vi "Oscilloscope.vi"() -> ()   [LabVIEW 2018]
uses:
  NetworkStream/NetworkStreamReceiverState.ctl
  Read and Save Files/VIstatus.ctl
  NetworkStream/NetworkStreamStateMachineVariable.ctl
  NetworkStream/NetworkStreamData.ctl
  Shared program Control/MasterStatus.ctl
  <vilib>/dex/Stream Element Allocation Mode.ctl
  Read and Save Files/RW_Protocols.lvlib
  NetworkStream/NetworkStream.lvlib
  Shared program Control/MySharedVariables.lvlib
  Tektronik3102/GageNetwork.lvlib
panel:
  out "size(s)":i32[](array[numeric])
  out "loop status":T1
  out "Sequence Number":i64
  out "sequence number":u64
  out "Session Hash":u64
  out "Network Stream State Indicator":T2
  in  "Save Loop acquire":bool
  out "error out 2":errorcluster
  in  "loop acquire":bool
  in  "Tab Control 2":enum32{"single acquire", "sequence acquire"}(tab)
  out "Waveform Graph":dbl[][](graph)
  out "Intensity Chart":dbl[][](graph)
  out "aquire time (ms)":u32
  out "current aquisition":T3
  in  "abort aquisition":bool
  out "Handle Cluster":T4
  out "Gage progess":string
  in  "aquire":bool
  in  "Stop Button":bool
  out "error out":errorcluster
  in  "Tab Control":T5(tab)
  in  "channels \nconfiguration":T6(array[cluster])=[{"Coupling"=0, "Differential Input"=FALSE, "Direct-to-ADC"=FALSE, "Range"=2000, "Impedance"=50, "DC Offset"=0}, {"Coupling"=0, "Differential Input"=FALSE, "Direct-to-ADC"=FALSE, "Range"=2000, "Impedance"=50, "DC Offset"=0}, {"Coupling"=0, "Differential Input"=FALSE, "Direct-to-ADC"=FALSE, "Range"=2000, "Impedance"=50, "DC Offset"=0}, {"Coupling"=0, "Differential Input"=FALSE, "Direct-to-ADC"=FALSE, "Range"=2000, "Impedance"=50, "DC Offset"=0}] {"Impedance" min=50 max=1000000 step=999950; "Coupling" items=["DC", "AC"]}
  in  "Continuous":bool
  in  "Trigger":T7={"Slope"=0, "Level"=0, "Source"=0, "External Range"=2000, "External Coupling"=0, "External"=FALSE, "Disable"=FALSE, "External Impedance"=1} {"External Impedance" items=["50 Ohm", "HiZ"]; "External Coupling" items=["DC", "AC"]; "External Range" min=2000 max=10000 step=8000; "Slope" items=["Rising", "Falling"]; "Level" min=-100 max=100; "Source" min=0 max=64 step=1}
  in  "Acquisition":T8={"Sample Rate"=1000000.0, "Clock mode"=enum."Internal", "Mode"=0, "post trigger"=8192.0, "Segment Size"=8192.0, "Trigger Timeout"=100000.0, "Trigger Holdoff"=0.0, "Trigger Delay"=0.0, "averaging "=1} {"Segment Size" min=256.0 step=128.0; "Trigger Holdoff" min=0.0 step=128.0; "Trigger Delay" min=0.0 step=128.0; "post trigger" min=256.0 step=128.0; "Mode" items=["Single", "Dual", "Quad", "Octal"]}
  in  "configure":bool
  in  "saving folder":path=path "D:/Data/Mai/test target/logfile"
  in  "file name":string
  out "System:":string
  out "system information":T9
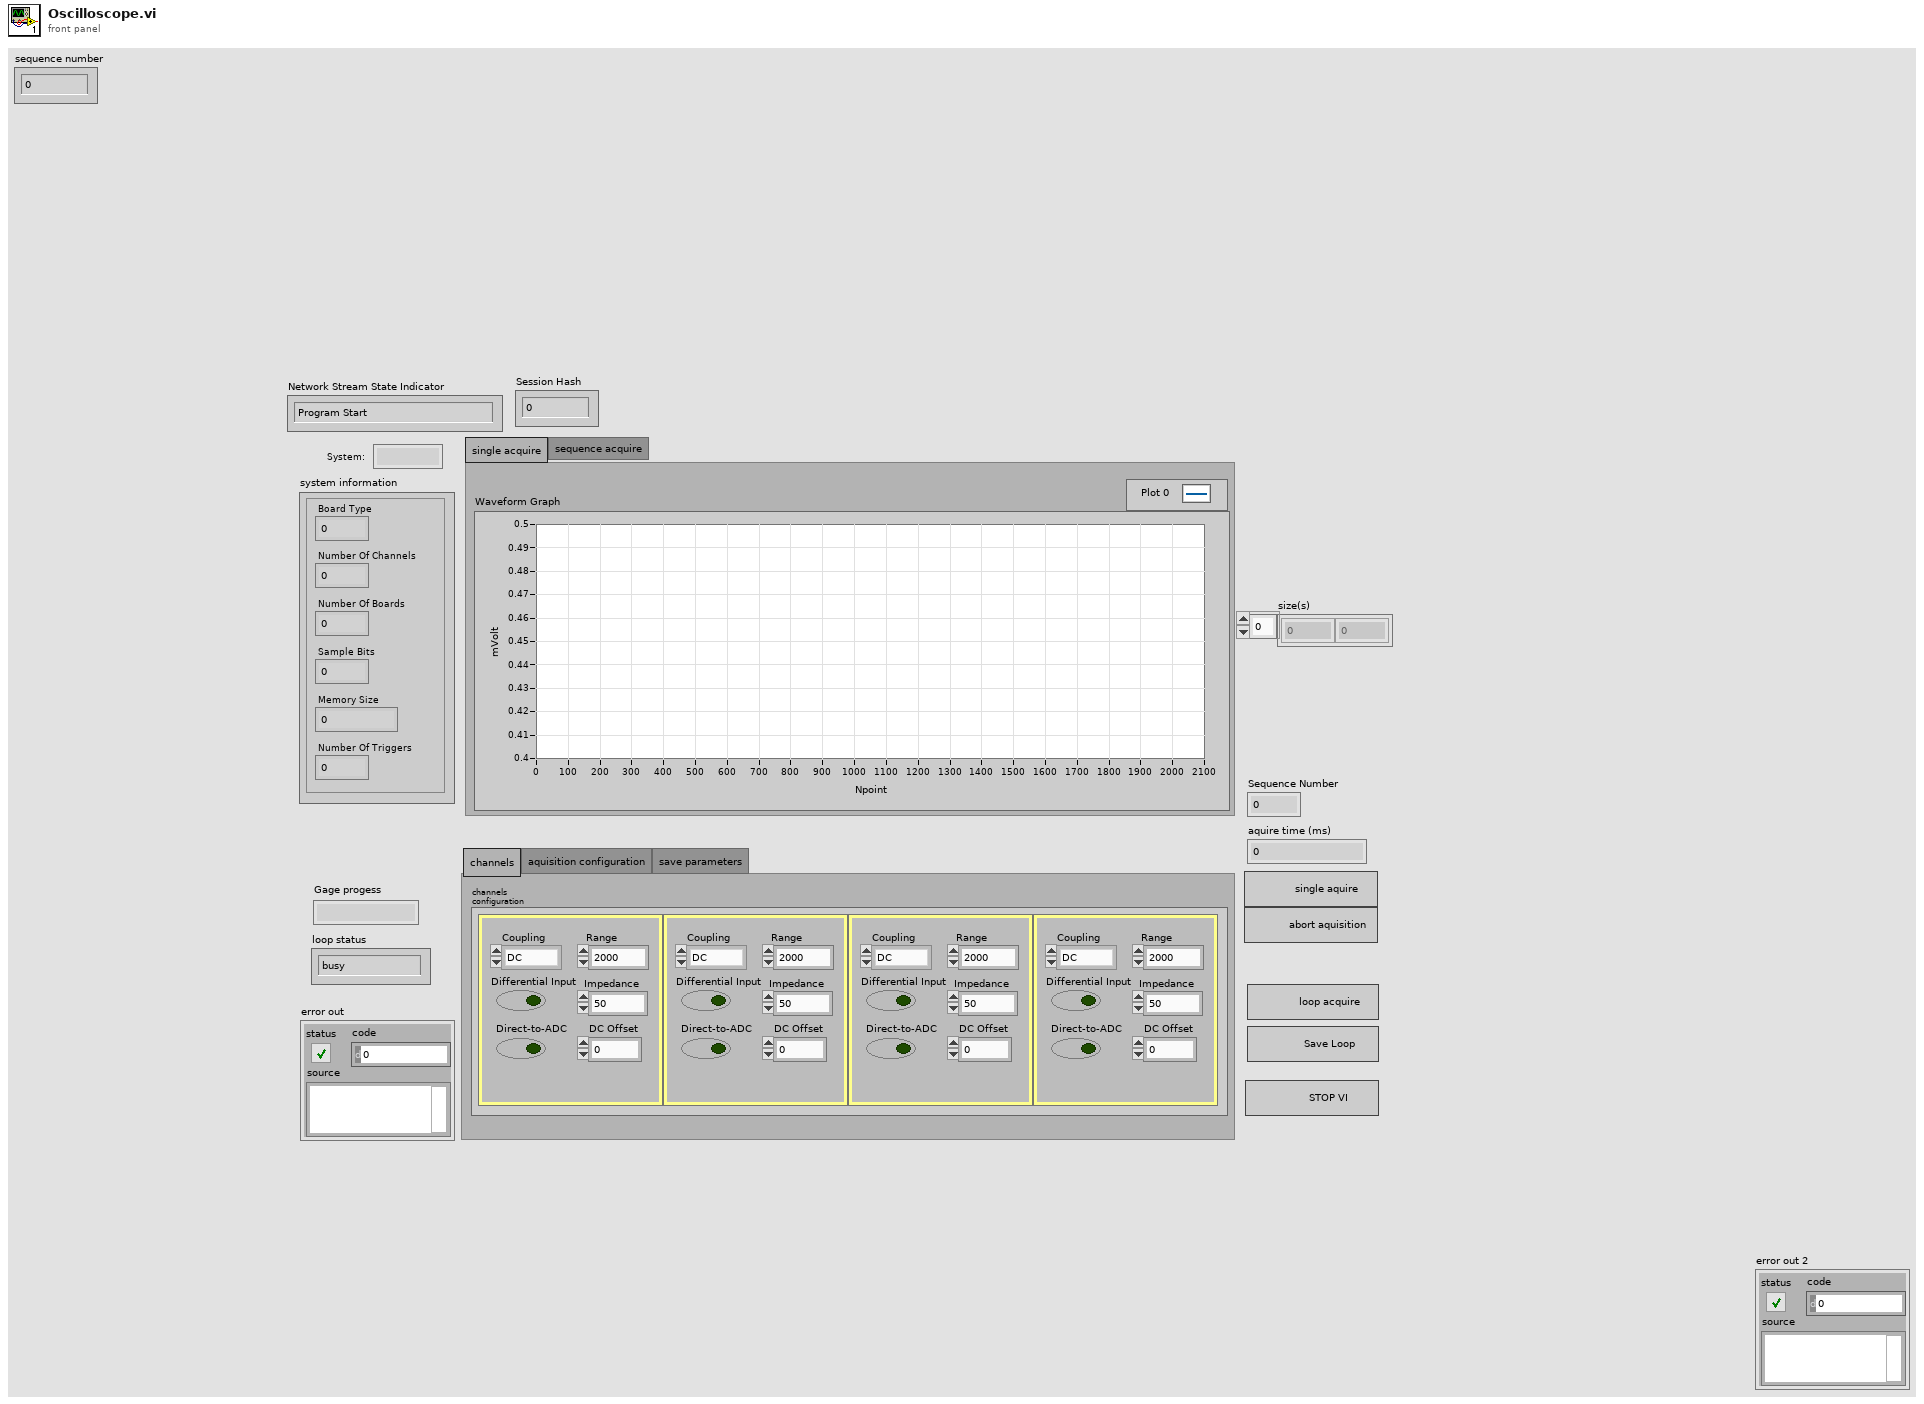
[diagram p1: front panel]
types:
  T1 = typedef "VIstatus.ctl" = enum16{"busy", "update config", "wait", "single acquire", "stop VI", "loop acquire"}
  T2 = typedef "NetworkStream.lvlib/NetworkStreamReceiverState.ctl" = enum16{"Program Start", "Waiting for connection", "Connected", "Connection lost", "Exit", "Unhandled Exception"}
  T3 = cluster{"Sample Rate":dbl, "Clock mode":enum16{"Internal", "External", "Reference"}, "Mode":u16, "post trigger":dbl, "Segment Size":dbl, "Trigger Timeout":dbl, "Trigger Holdoff":dbl, "Trigger Delay":dbl, "number of records":u32}
  T4 = cluster{"Handle":u32, "Sample size":u32, "Resolution":i32, "Offset":i32, "Channels":u32, "Boards":u32}
  T5 = enum32{"channels", "aquisition configuration", "save parameters"}
  T6 = cluster{"Coupling":u16, "Differential Input":bool, "Direct-to-ADC":bool, "Range":u32, "Impedance":u32, "DC Offset":i32}[]
  T7 = cluster{"Slope":u16, "Level":i32, "Source":i32, "External Range":u32, "External Coupling":u16, "External":bool, "Disable":bool, "External Impedance":u16}
  T8 = cluster{"Sample Rate":dbl, "Clock mode":enum16{"Internal", "External", "Reference"}, "Mode":u16, "post trigger":dbl, "Segment Size":dbl, "Trigger Timeout":dbl, "Trigger Holdoff":dbl, "Trigger Delay":dbl, "averaging ":u32}
  T9 = cluster{"Memory Size":dbl, "Board Type":u32, "Number Of Channels":u32, "Number Of Boards":u32, "Sample Bits":u32, "Number Of Triggers":u32}
  T10 = typedef "MySharedVariables.lvlib/MasterStatus.ctl" = cluster{"Camera done":bool, "Tektronik done":bool, "Motors done":bool, "Gage done":bool}[]
  T11 = typedef "NetworkStream.lvlib/NetworkStreamData.ctl" = cluster{"Command/Status":string, "Data":variant, "Session Hash":u64, "Sequence Number":u64}
  T12 = typedef "NetworkStream.lvlib/NetworkStreamStateMachineVariable.ctl" = cluster{"Network Stream Reader Endpoint":refnum<k21>, "Last Received Sequence Number":u64}
  T13 = enum8{"Enabled", "Disabled", "Disabled and Grayed Out"}
  T14 = typedef "Stream Element Allocation Mode.ctl" = u32
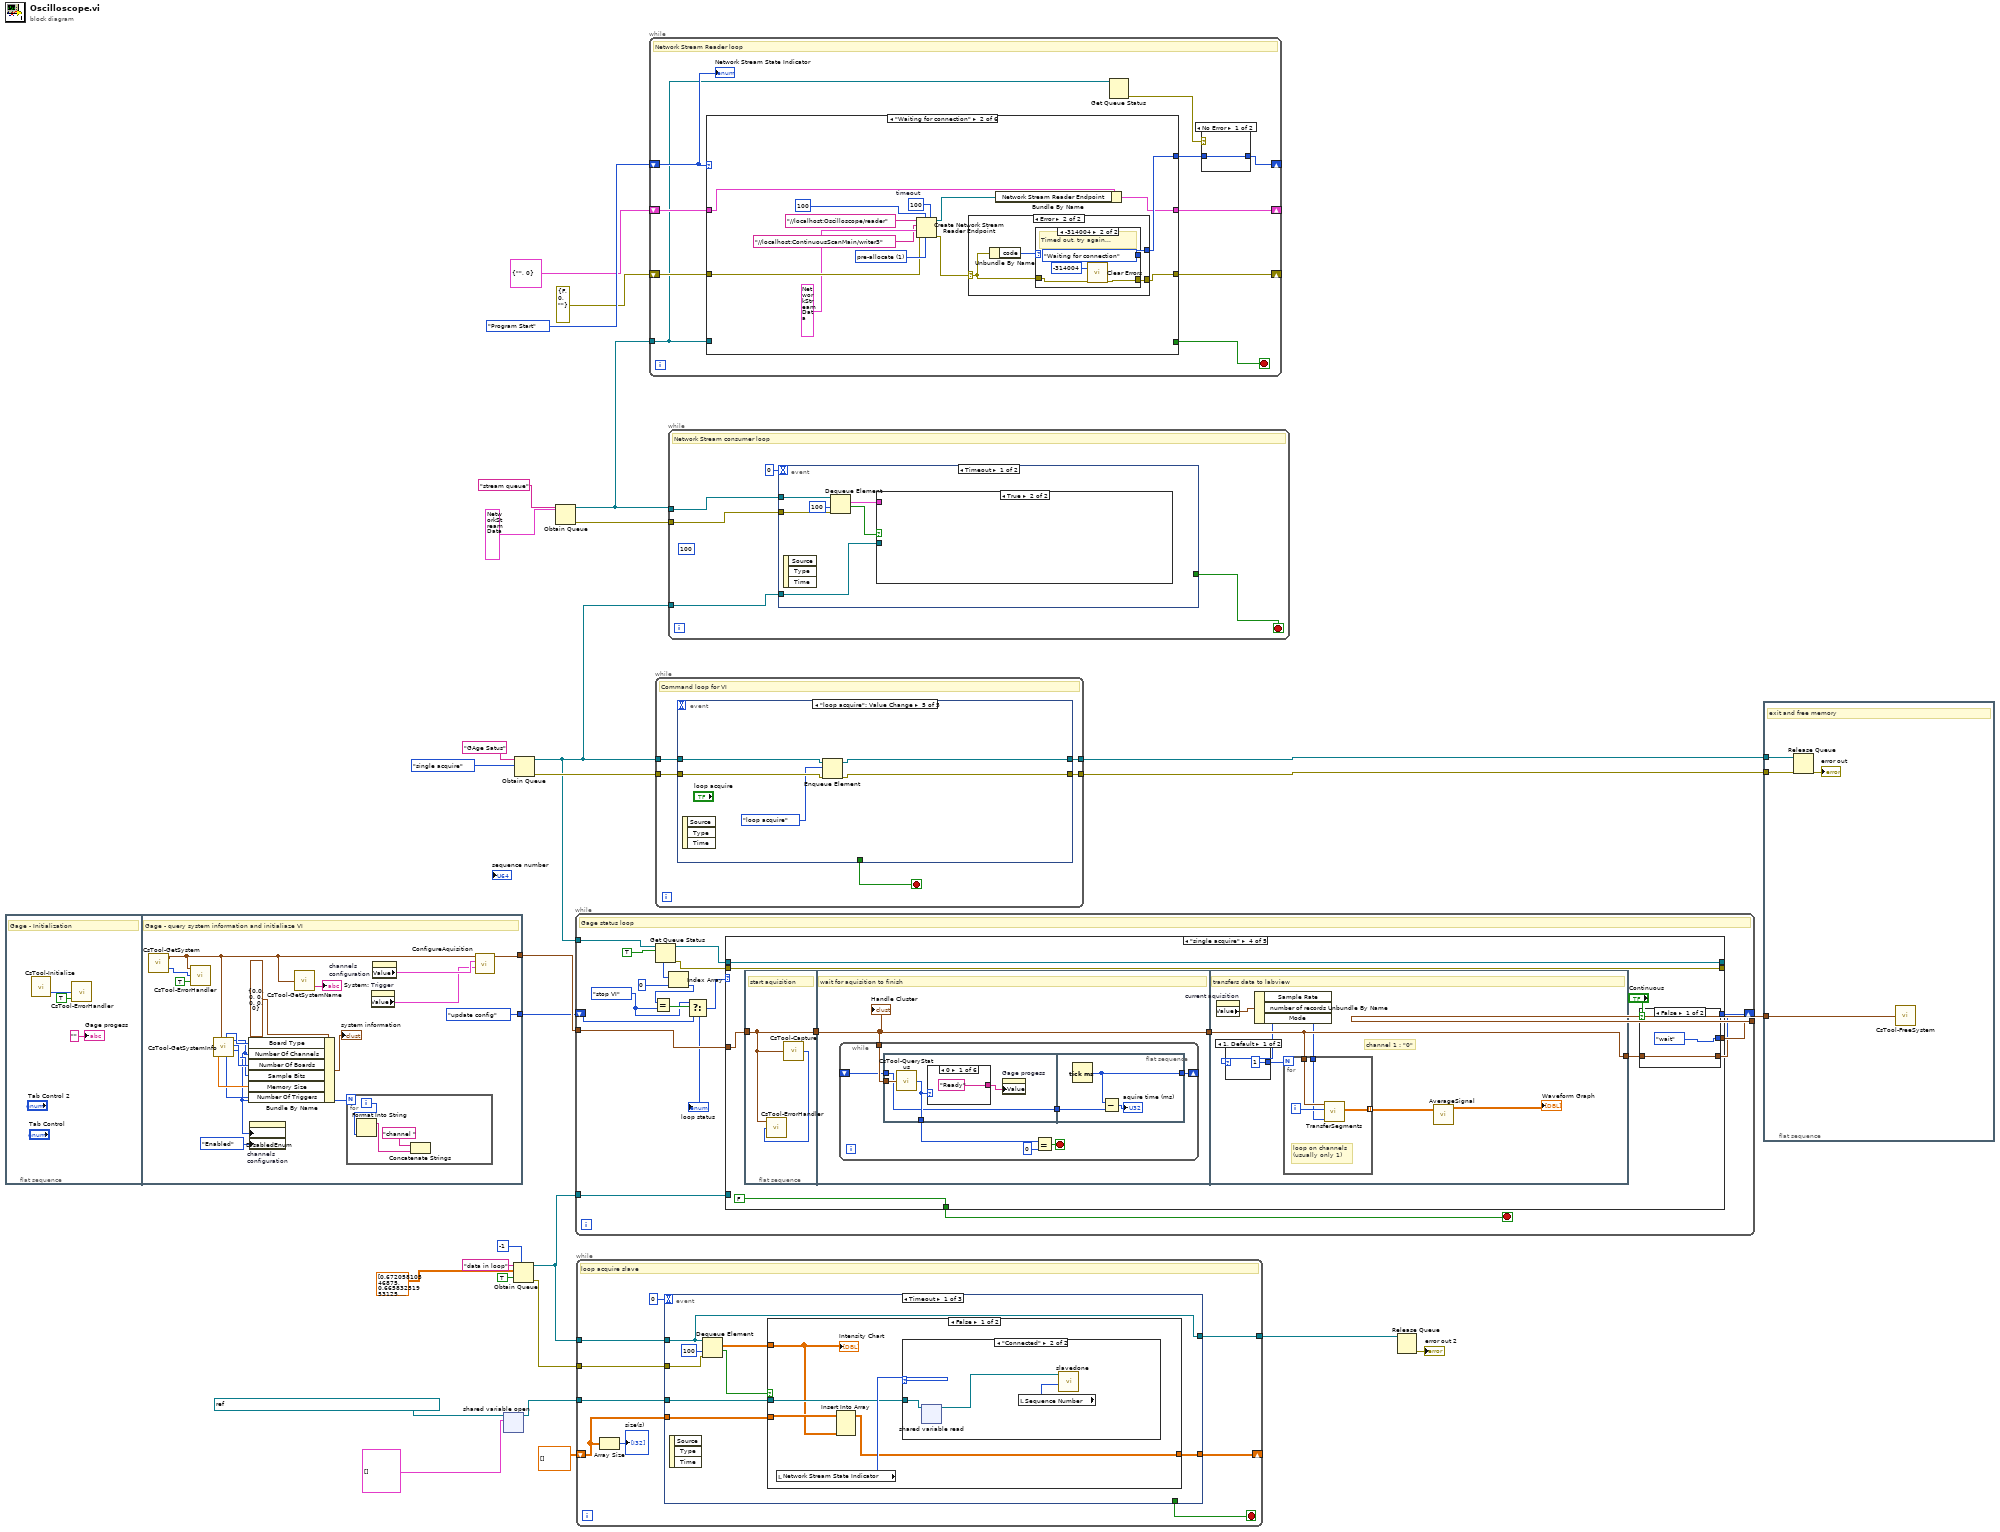
[diagram p0: block diagram]
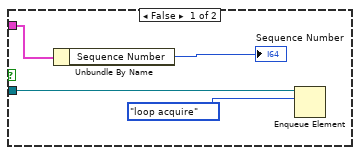
[diagram p2: hidden frame]
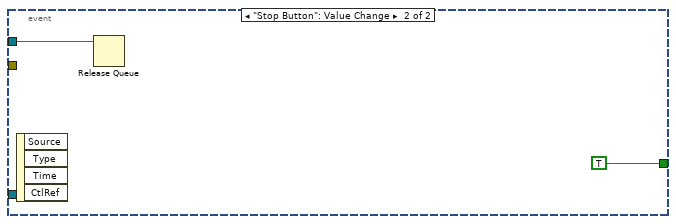
[diagram p3: hidden frame]
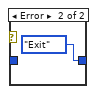
[diagram p4: hidden frame]
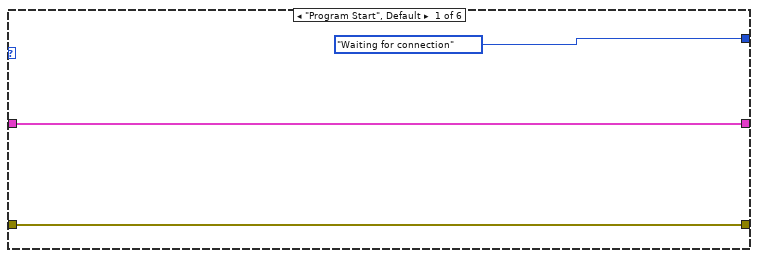
[diagram p5: hidden frame]
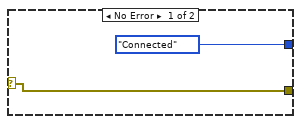
[diagram p6: hidden frame]
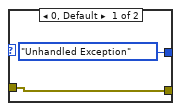
[diagram p7: hidden frame]
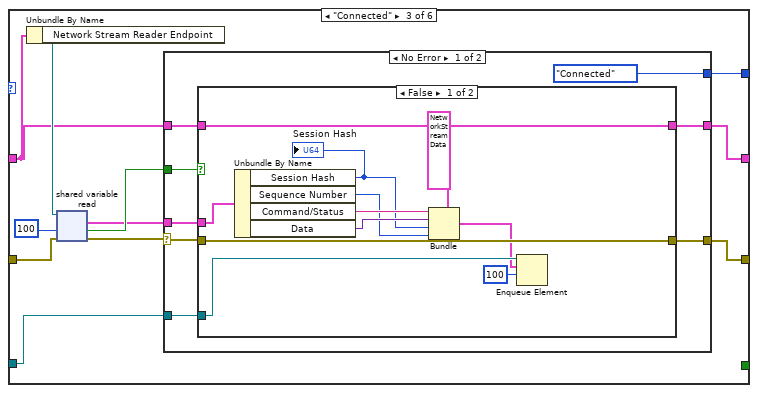
[diagram p8: hidden frame]
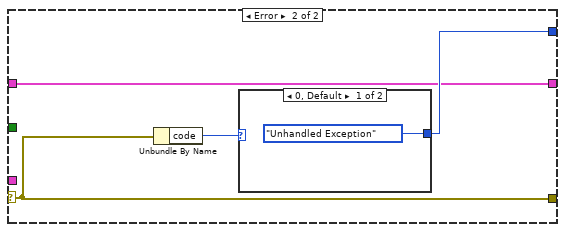
[diagram p10: hidden frame]
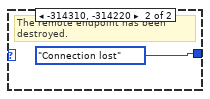
[diagram p11: hidden frame]
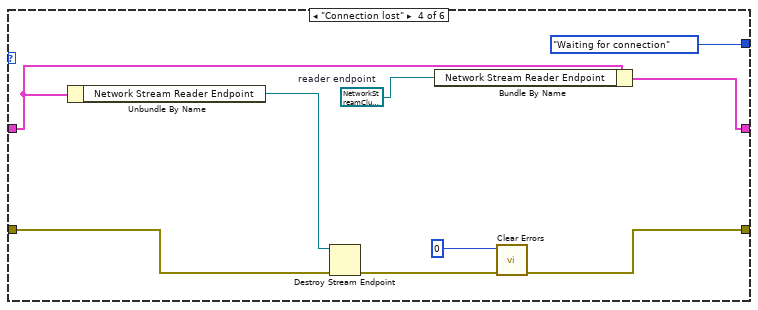
[diagram p12: hidden frame]
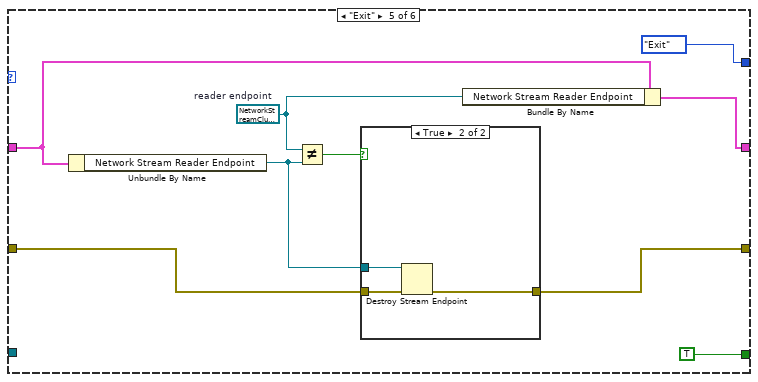
[diagram p13: hidden frame]
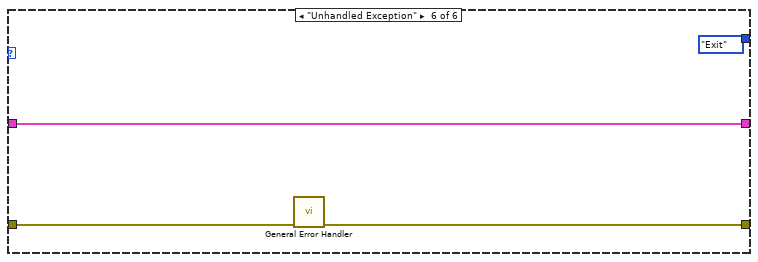
[diagram p15: hidden frame]
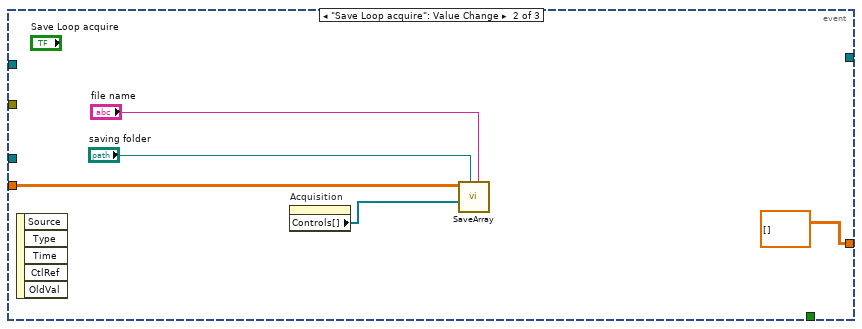
[diagram p18: hidden frame]
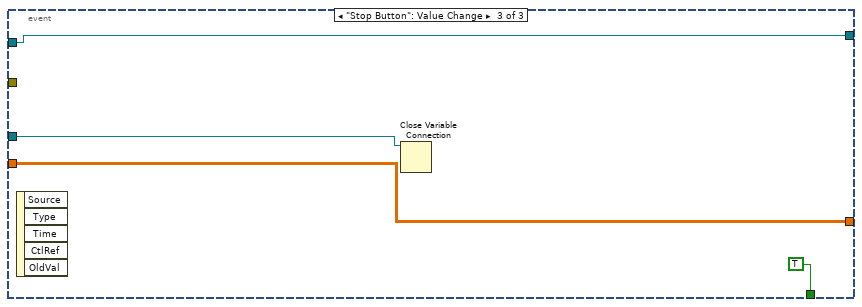
[diagram p19: hidden frame]
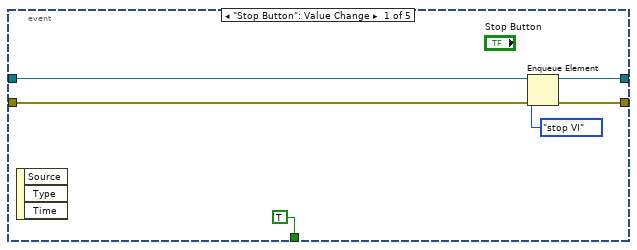
[diagram p20: hidden frame]
diagram:
  n1 = flat-sequence {
    tunnel: [w34] -> w28
    tunnel: [VIstatus."update config" ("VI status")] -> w22
    frame #0 {
      # "Gage - Initialization"
      n2 = call <userlib>:"CsTool-Initialize.vi"() -> ("Error Code"=w31:i32)  [unwired: 1 out]
      n3 = call <userlib>:"CsTool-ErrorHandler.vi"("StopOnError (true)"=TRUE, "Error Code"=w31) -> ()  [unwired: 1 in, 1 out]
      "Gage progess" <- "" ("Gage progess")
    }
    frame #1 {
      # "Gage - query system information and initialiaze VI"
      n4 = call <userlib>:"CsTool-GetSystem.vi"() -> ("Error Code"=w36:i32, "Handle Cluster"=w35:T4)  [unwired: 4 in]
      n5 = call <userlib>:"CsTool-ErrorHandler.vi"("StopOnError (true)"=TRUE, "Error Code"=w36, "Handle Cluster"=w35) -> ()  [unwired: 1 out]
      n6 = call <userlib>:"CsTool-GetSystemInfo.vi"("Handle Cluster"=w35) -> ("Memory Size"=w45:dbl, "Board Type"=w48:u32, "Number Of Triggers"=w43:u32, "Number Of Channels"=w39:u32, "Number Of Boards"=w47:u32, "Sample Bits"=w46:u32)  [unwired: 1 out]
      n7 = Bundle By Name(cluster=T9 {"Memory Size"=0.0, "Board Type"=0, "Number Of Channels"=0, "Number Of Boards"=0, "Sample Bits"=0, "Number Of Triggers"=0} ("system information"), "Board Type"=w48, "Number Of Channels"=w39, "Number Of Boards"=w47, "Sample Bits"=w46, "Memory Size"=w45, "Number Of Triggers"=w43) -> (→"system information":T9)
      n8 = property on="channels \nconfiguration" class="Arr (strict)"("Number of Columns"=w39, "DisabledEnum"=T13."Enabled" ("Disabled")) -> ()  [unwired: 2 in, 2 out]
      n9 = call <userlib>:"CsTool-GetSystemName.vi"("Handle Cluster"=w35) -> ("System Name"=→"System:":string)  [unwired: 1 out]
      n10 = for {
        N: w39 -> [_]
        i -> [w50]
        n11 = Format Into String(w50) -> (resulting string=w49:string)  [unwired: 3 in, 1 out]
        n12 = Concatenate Strings("channel ", w49) -> ()  [unwired: 1 out]
      }
      n13 = property on="Trigger" class="Clust (strict)"() -> ("Value"=w32:T7)  [unwired: 2 in, 2 out]
      n14 = property on="channels \nconfiguration" class="Arr (strict)"() -> ("Value"=w33:T6)  [unwired: 2 in, 2 out]
      n15 = call "ConfigureAquisition.vi"("Trigger"=w32, "channels configuration"=w33, "Handle Cluster"=w35) -> ("Handle Cluster 2"=w34:T4)  [unwired: 7 in, 1 out]
    }
  }
  n16 = shared-variable-open(refnum<k21> "ni.var.psp://localhost/MySharedVariables/MasterStatusShared" ("shared variable refnum in"), T10 [] ("MasterStatusShared")) -> (w5:refnum<k21>)  [unwired: 2 in, 1 out]
  n17 = Obtain Queue(max queue size (-1, unlimited)=-1, name (unnamed)="data in loop", element data type=dbl[][] [[0.67205810546875, 0.66583251953125, 0.68377685546875, 0.69293212890625, 0.68572998046875, 0.69537353515625, 0.67730712890625, 0.66571044921875, 0.70660400390625, 0.65374755859375, 0.68536376953125, 0.66754150390625, 0.68145751953125, 0.64459228515625, 0.67388916015625, 0.69647216796875, 0.70062255859375, 0.69512939453125, 0.70367431640625, 0.69598388671875, 0.70928955078125, 0.67633056640625, 0.67938232421875, 0.68768310546875, 0.67755126953125, 0.71136474609375, 0.69256591796875, 0.71734619140625, 0.69085693359375, 0.67864990234375, 0.67864990234375, 0.70330810546875, 0.68621826171875, 0.69439697265625, 0.68878173828125, 0.71185302734375, 0.67327880859375, 0.69573974609375, 0.70440673828125, 0.69439697265625, 0.65728759765625, 0.68768310546875, 0.68060302734375, 0.67950439453125, 0.67144775390625, 0.69793701171875, 0.69317626953125, 0.67437744140625, 0.69708251953125, 0.66766357421875, 0.69097900390625, 0.67584228515625, 0.68902587890625, 0.66314697265625, 0.68804931640625, 0.68328857421875, 0.68353271484375, 0.68463134765625, 0.69012451171875, 0.69512939453125, 0.71612548828125, 0.66802978515625, 0.67279052734375, 0.67938232421875, 0.67169189453125, 0.67864990234375, 0.67254638671875, 0.65594482421875, 0.66168212890625, 0.67816162109375, 0.66497802734375, 0.70281982421875, 0.69757080078125, 0.69317626953125, 0.70562744140625, 0.68328857421875, 0.69195556640625, 0.66729736328125, 0.69720458984375, 0.66546630859375, 0.66790771484375, 0.68438720703125, 0.68560791015625, 0.69561767578125, 0.67742919921875, 0.71185302734375, 0.68328857421875, 0.67999267578125, 0.68218994140625, 0.69134521484375, 0.66973876953125, 0.69305419921875, 0.69232177734375, 0.71600341796875, 0.72003173828125, 0.71551513671875, 0.69464111328125, 0.70843505859375, 0.71173095703125, 0.69061279296875, 0.70538330078125, 0.68231201171875, 0.69183349609375, 0.68096923828125, 0.70819091796875, 0.68145751953125, 0.68829345703125, 0.74554443359375, 0.69573974609375, 0.70452880859375, 0.70526123046875, 0.71307373046875, 0.69903564453125, 0.67230224609375, 0.65777587890625, 0.63885498046875, 0.69317626953125, 0.69305419921875, 0.67791748046875, 0.69940185546875, 0.67657470703125, 0.68548583984375, 0.68011474609375, 0.68231201171875, 0.70660400390625, 0.69488525390625, 0.68829345703125, 0.68170166015625, 0.71136474609375, 0.66143798828125, 0.66741943359375, 0.67852783203125, 0.69195556640625, 0.68084716796875, 0.67864990234375, 0.71563720703125, 0.68072509765625, 0.69354248046875, 0.67108154296875, 0.68450927734375, 0.67974853515625, 0.68695068359375, 0.69989013671875, 0.69744873046875, 0.68853759765625, 0.68609619140625, 0.68292236328125, 0.68902587890625, 0.68865966796875, 0.66741943359375, 0.68670654296875, 0.69732666015625, 0.67071533203125, 0.69500732421875, 0.66937255859375, 0.72015380859375, 0.69427490234375, 0.69158935546875, 0.69268798828125, 0.68914794921875, 0.67327880859375, 0.67694091796875, 0.69110107421875, 0.69488525390625, 0.68499755859375, 0.70343017578125, 0.71832275390625, 0.69976806640625, 0.66839599609375, 0.68365478515625, 0.68048095703125, 0.70635986328125, 0.70892333984375, 0.65777587890625, 0.70513916015625, 0.70623779296875, 0.70159912109375, 0.72332763671875, 0.69586181640625, 0.69879150390625, 0.68218994140625, 0.70086669921875, 0.66961669921875, 0.66888427734375, 0.69000244140625, 0.69488525390625, 0.70513916015625, 0.68231201171875, 0.70172119140625, 0.69964599609375, 0.69830322265625, 0.67071533203125, 0.68377685546875, 0.70892333984375, 0.69036865234375, 0.67462158203125, 0.67864990234375, 0.68023681640625, 0.68365478515625, 0.69769287109375, 0.69732666015625, 0.69732666015625, 0.67547607421875, 0.69146728515625, 0.69366455078125, 0.68597412109375, 0.70428466796875, 0.69268798828125, 0.70904541015625, 0.71685791015625, 0.69891357421875, 0.72406005859375, 0.71600341796875, 0.71539306640625, 0.69219970703125, 0.73358154296875, 0.69818115234375, 0.69476318359375, 0.70721435546875, 0.71002197265625, 0.71771240234375, 0.73626708984375, 0.70855712890625, 0.72491455078125, 0.71942138671875, 0.73150634765625, 0.72235107421875, 0.72967529296875, 0.71417236328125, 0.71905517578125, 0.72747802734375, 0.75152587890625, 0.73834228515625, 0.74871826171875, 0.73651123046875, 0.73211669921875, 0.74188232421875, 0.73760986328125, 0.75921630859375, 0.74261474609375, 0.74737548828125, 0.76812744140625, 0.76068115234375, 0.75201416015625, 0.78057861328125, 0.77667236328125, 0.80999755859375, 0.79571533203125, 0.79644775390625, 0.77264404296875, 0.78887939453125, 0.79107666015625, 0.77362060546875, 0.78387451171875, 0.81219482421875, 0.75714111328125, 0.79132080078125, 0.80279541015625, 0.81317138671875, 0.81256103515625, 0.80706787109375, 0.81964111328125, 0.81329345703125, 0.79327392578125, 0.84307861328125, 0.82635498046875, 0.84893798828125, 0.82000732421875, 0.85174560546875, 0.84136962890625, 0.86309814453125, 0.85516357421875, 0.84039306640625, 0.85687255859375, 0.83758544921875, 0.88421630859375, 0.86614990234375, 0.87823486328125, 0.87664794921875, 0.87359619140625, 0.88726806640625, 0.87091064453125, 0.87872314453125, 0.87896728515625, 0.87933349609375, 0.92132568359375, 0.90325927734375, 0.88702392578125, 0.91070556640625, 0.91729736328125, 0.89215087890625, 0.90704345703125, 0.93218994140625, 0.92193603515625, 0.94598388671875, 0.91278076171875, 0.92974853515625, 0.96575927734375, 0.93853759765625, 0.91644287109375, 0.93865966796875, 0.90509033203125, 0.92657470703125, 0.94488525390625, 0.92913818359375, 0.92315673828125, 0.94976806640625, 0.98455810546875, 0.95599365234375, 0.93048095703125, 0.95574951171875, 0.94989013671875, 0.95928955078125, 0.97015380859375, 0.98126220703125, 0.98114013671875, 0.95977783203125, 0.98699951171875, 0.92877197265625, 0.96173095703125, 0.98211669921875, 0.97674560546875, 0.96258544921875, 0.96453857421875, 0.95953369140625, 1.00152587890625, 0.98919677734375, 0.99847412109375, 0.94525146484375, 0.96490478515625, 0.96734619140625, 0.96392822265625, 0.99334716796875, 0.98272705078125, 0.97833251953125, 0.95123291015625, 0.98236083984375, 0.99554443359375, 0.96380615234375, 0.95111083984375, 0.97149658203125, 0.97174072265625, 0.92669677734375, 0.96429443359375, 0.95562744140625, 0.96539306640625, 0.95916748046875, 0.96917724609375, 0.98541259765625, 0.97479248046875, 0.94769287109375, 0.98883056640625, 0.97015380859375, 0.96441650390625, 0.96038818359375, 0.97015380859375, 0.94378662109375, 0.92803955078125, 0.95672607421875, 0.95916748046875, 0.93878173828125, 0.97271728515625, 0.94793701171875, 0.97796630859375, 0.96478271484375, 0.94036865234375, 0.98773193359375, 0.96160888671875, 0.97100830078125, 0.99053955078125, 0.92620849609375, 0.97039794921875, 0.97113037109375, 0.97808837890625, 0.95343017578125, 0.94866943359375, 0.96319580078125, 0.96209716796875, 0.93402099609375, 0.96221923828125, 0.97943115234375, 0.93878173828125, 1.00238037109375, 0.97015380859375, 0.99224853515625, 0.95147705078125, 0.96881103515625, 0.98223876953125, 0.95770263671875, 0.96453857421875, 0.96978759765625, 0.97271728515625, 0.95660400390625, 0.97393798828125, 0.96685791015625, 0.95184326171875, 0.99078369140625, 0.98785400390625, 0.98712158203125, 0.95355224609375, 0.97198486328125, 0.96429443359375, 0.94708251953125, 0.97845458984375, 0.97161865234375, 0.92816162109375, 1.00177001953125, 0.96087646484375, 0.97576904296875, 0.96197509765625, 0.95599365234375, 0.97113037109375, 0.96160888671875, 0.96466064453125, 0.98236083984375, 0.96697998046875, 0.93646240234375, 0.94842529296875, 0.96136474609375, 0.95819091796875, 0.95404052734375, 0.94207763671875, 0.95074462890625, 0.95513916015625, 0.95941162109375, 0.97296142578125, 0.97430419921875, 0.97674560546875, 0.96246337890625, 0.94903564453125, 0.95831298828125, 0.97821044921875, 0.95867919921875, 0.94378662109375, 0.94171142578125, 0.93243408203125, 0.94476318359375, 0.98248291015625, 0.97076416015625, 0.96441650390625, 0.99456787109375, 0.93365478515625, 0.96527099609375, 0.95062255859375, 0.97711181640625, 0.96844482421875, 0.96527099609375, 0.97747802734375, 0.97186279296875, 0.95953369140625, 0.95599365234375, 0.95526123046875, 0.98223876953125, 0.97894287109375, 0.98297119140625, 0.97064208984375, 0.95782470703125, 0.99310302734375, 0.95526123046875, 0.99835205078125, 0.97686767578125, 0.98382568359375, 0.95709228515625, 0.97088623046875, 0.99053955078125, 0.97821044921875, 0.99017333984375, 0.95477294921875, 0.98223876953125, 0.96527099609375, 0.97503662109375, 0.96722412109375, 0.98248291015625, 0.95233154296875, 0.99652099609375, 0.97662353515625, 0.97454833984375, 0.98162841796875, 0.94573974609375, 0.96868896484375, 0.97406005859375, 0.94122314453125, 0.97186279296875, 0.93426513671875, 0.96441650390625, 0.97344970703125, 0.95550537109375, 0.93377685546875, 0.96160888671875, 0.96441650390625, 0.96160888671875, 0.98077392578125, 0.93817138671875, 0.95037841796875, 0.98699951171875, 0.95965576171875, 0.94635009765625, 0.97955322265625, 0.96124267578125, 0.98175048828125, 0.94671630859375, 0.98040771484375, 0.96856689453125, 0.95318603515625, 0.95660400390625, 0.93865966796875, 0.95489501953125, 0.93988037109375, 0.95343017578125, 0.93048095703125, 0.96710205078125, 0.97491455078125, 0.93585205078125, 0.98309326171875, 0.94012451171875, 0.98040771484375, 0.96466064453125, 0.96551513671875, 0.93988037109375, 0.93304443359375, 0.94183349609375, 0.93011474609375, 0.92449951171875, 0.95391845703125, 0.94024658203125, 0.95831298828125, 0.94305419921875, 0.96490478515625, 0.97955322265625, 0.94415283203125, 0.96368408203125, 0.96612548828125, 0.97308349609375, 0.95062255859375, 0.96002197265625, 0.95135498046875, 0.96600341796875, 0.97735595703125, 0.95782470703125, 0.97418212890625, 0.96026611328125, 0.96319580078125, 0.94842529296875, 0.95599365234375, 0.95428466796875, 0.97442626953125, 0.95306396484375, 0.95513916015625, 0.94537353515625, 0.93585205078125, 0.95318603515625, 0.97955322265625, 0.95489501953125, 0.96392822265625, 0.95892333984375, 0.95281982421875, 0.95721435546875, 0.97344970703125, 0.96514892578125, 0.96099853515625, 0.93988037109375, 0.93731689453125, 0.94049072265625, 0.96246337890625, 0.94464111328125, 0.95538330078125, 0.95269775390625, 0.96563720703125, 0.94964599609375, 0.95745849609375, 0.92498779296875, 0.96954345703125, 0.95281982421875, 0.96417236328125, 0.91778564453125, 0.97100830078125, 0.95208740234375, 0.94927978515625, 0.92572021484375, 0.92340087890625, 0.94244384765625, 0.95758056640625, 0.95159912109375, 0.94146728515625, 0.95159912109375, 0.95111083984375, 0.92437744140625, 0.96600341796875, 0.93328857421875, 0.93182373046875, 0.94158935546875, 0.95574951171875, 0.96392822265625, 0.93109130859375, 0.95343017578125, 0.94525146484375, 0.96942138671875, 0.96368408203125, 0.97198486328125, 0.95050048828125, 0.95196533203125, 0.96209716796875, 0.97637939453125, 0.98516845703125, 0.99761962890625, 0.96417236328125, 0.98431396484375, 0.94561767578125, 0.96307373046875, 0.94830322265625, 0.95941162109375, 0.96331787109375, 0.98992919921875, 0.95855712890625, 0.97137451171875, 0.95562744140625, 0.98028564453125, 0.98577880859375, 0.95208740234375, 0.95758056640625, 0.97296142578125, 0.95928955078125, 0.95526123046875, 0.93048095703125, 0.96136474609375, 0.95294189453125, 0.97113037109375, 0.96881103515625, 0.97308349609375, 0.97003173828125, 0.94012451171875, 0.95526123046875, 0.94622802734375, 0.97613525390625, 0.95245361328125, 0.95281982421875, 0.95623779296875, 0.97052001953125, 0.95867919921875, 0.96954345703125, 0.96319580078125, 0.95245361328125, 0.95184326171875, 0.95379638671875, 0.96954345703125, 0.98675537109375, 0.94561767578125, 0.96246337890625, 0.95074462890625, 0.94488525390625, 0.97027587890625, 0.95782470703125, 0.97882080078125, 0.96759033203125, 0.95965576171875, 0.96380615234375, 0.94915771484375, 0.96002197265625, 0.98736572265625, 0.96624755859375, 0.97698974609375, 0.95587158203125, 0.91790771484375, 0.96221923828125, 0.95465087890625, 0.97711181640625, 0.95684814453125, 0.97637939453125, 0.94842529296875, 0.97967529296875, 0.96759033203125, 0.96160888671875, 0.95477294921875, 0.96112060546875, 0.97271728515625, 0.98028564453125, 0.97186279296875, 0.97943115234375, 0.97772216796875, 0.96356201171875, 1.00982666015625, 0.98358154296875, 0.94158935546875, 0.96844482421875, 0.95489501953125, 0.96258544921875, 0.99676513671875, 0.98907470703125, 0.97943115234375, 0.96990966796875, 0.95294189453125, 0.95172119140625, 0.97979736328125, 0.95428466796875, 0.96942138671875, 0.94366455078125, 0.95611572265625, 0.96417236328125, 0.95709228515625, 0.94940185546875, 0.93768310546875, 0.95599365234375, 0.94390869140625, 0.97479248046875, 0.92840576171875, 0.96881103515625, 0.94464111328125, 0.96856689453125, 0.95843505859375, 0.95672607421875, 0.96258544921875, 0.93963623046875, 0.93341064453125, 0.95452880859375, 0.94805908203125, 0.98101806640625, 0.98834228515625, 0.98468017578125, 0.94525146484375, 0.99432373046875, 0.95513916015625, 0.95001220703125, 0.97552490234375, 0.96441650390625, 0.94915771484375, 0.95306396484375, 0.96844482421875, 0.96002197265625, 0.95758056640625, 0.94061279296875, 0.94525146484375, 0.96490478515625, 0.97808837890625, 0.96026611328125, 0.94488525390625, 0.95404052734375, 0.96844482421875, 0.94512939453125, 0.94854736328125, 0.98077392578125, 0.98638916015625, 0.96893310546875, 0.97723388671875, 0.95587158203125, 0.97064208984375, 0.96343994140625, 0.98626708984375, 0.96051025390625, 0.97564697265625, 0.97344970703125, 0.95660400390625, 0.96258544921875, 0.96942138671875, 0.96295166015625, 0.97003173828125, 0.94732666015625, 0.98614501953125, 0.97503662109375, 0.99761962890625, 0.96893310546875, 0.96295166015625, 0.96954345703125, 0.94403076171875, 0.94635009765625, 0.97222900390625, 0.96246337890625, 0.95269775390625, 0.96075439453125, 0.94293212890625, 0.96258544921875, 0.96173095703125, 0.96185302734375, 0.95062255859375, 0.94573974609375, 0.92779541015625, 0.93914794921875, 0.96478271484375, 0.96514892578125, 0.95050048828125, 0.96502685546875, 0.95977783203125, 0.95538330078125, 0.94866943359375, 0.95526123046875, 0.96661376953125, 0.94842529296875, 0.97247314453125, 0.92144775390625, 0.98089599609375, 0.95904541015625, 0.98663330078125, 0.96966552734375, 0.94366455078125, 0.97723388671875, 0.94195556640625, 0.99285888671875, 0.96600341796875, 0.97613525390625, 0.95989990234375, 0.96185302734375, 0.96417236328125, 0.95465087890625, 0.96160888671875, 0.96759033203125, 0.94549560546875, 0.93731689453125, 0.96856689453125, 0.97113037109375, 0.93853759765625, 0.93853759765625, 0.95526123046875, 0.94024658203125, 0.94989013671875, 0.96820068359375, 0.94244384765625, 0.94842529296875, 0.95782470703125, 0.96795654296875, 0.94696044921875, 0.95831298828125, 0.96417236328125, 0.95806884765625, 0.93389892578125, 0.94134521484375, 0.94610595703125, 0.98455810546875, 0.95391845703125, 0.96112060546875, 0.97039794921875, 0.92706298828125, 0.93145751953125, 0.94024658203125, 0.95257568359375, 0.95172119140625, 0.91937255859375, 0.92437744140625, 0.93304443359375, 0.92254638671875, 0.91912841796875, 0.91143798828125, 0.91217041015625, 0.93792724609375, 0.92694091796875, 0.92254638671875, 0.90264892578125, 0.88531494140625, 0.90887451171875, 0.88360595703125, 0.88983154296875, 0.87396240234375, 0.88873291015625, 0.85113525390625, 0.87542724609375, 0.86114501953125, 0.88116455078125, 0.85003662109375, 0.85418701171875, 0.85516357421875, 0.84515380859375, 0.84368896484375, 0.85552978515625, 0.84429931640625, 0.83819580078125, 0.83306884765625, 0.82757568359375, 0.82427978515625, 0.80950927734375, 0.79302978515625, 0.82244873046875, 0.81781005859375, 0.77728271484375, 0.79522705078125, 0.80267333984375, 0.78692626953125, 0.77752685546875, 0.80206298828125, 0.78692626953125, 0.75726318359375, 0.77056884765625, 0.76263427734375, 0.76629638671875, 0.74371337890625, 0.74908447265625, 0.73919677734375, 0.76641845703125, 0.73651123046875, 0.77386474609375, 0.72393798828125, 0.75811767578125, 0.75860595703125, 0.74737548828125, 0.75042724609375, 0.73040771484375, 0.76617431640625, 0.71612548828125, 0.74774169921875, 0.74578857421875, 0.74420166015625, 0.72747802734375, 0.72906494140625, 0.72064208984375, 0.74591064453125, 0.71429443359375, 0.73394775390625, 0.74212646484375, 0.74188232421875, 0.76300048828125, 0.73211669921875, 0.69561767578125, 0.70489501953125, 0.69903564453125, 0.70477294921875, 0.69866943359375, 0.70526123046875, 0.72650146484375, 0.73138427734375, 0.69207763671875, 0.72100830078125, 0.69134521484375, 0.69183349609375, 0.69464111328125, 0.68670654296875, 0.71307373046875, 0.70965576171875, 0.70758056640625, 0.72015380859375, 0.70916748046875, 0.67706298828125, 0.70379638671875, 0.68963623046875, 0.70928955078125, 0.66400146484375, 0.71038818359375, 0.67877197265625, 0.67169189453125, 0.68975830078125, 0.67303466796875, 0.68621826171875, 0.67315673828125, 0.70574951171875, 0.70098876953125, 0.68853759765625, 0.69342041015625, 0.68792724609375, 0.70867919921875, 0.66180419921875, 0.69866943359375, 0.69146728515625, 0.69342041015625, 0.69183349609375, 0.71929931640625, 0.66522216796875, 0.71356201171875, 0.65948486328125, 0.68109130859375, 0.71002197265625, 0.69024658203125, 0.71978759765625, 0.68560791015625, 0.67340087890625, 0.69610595703125, 0.68585205078125, 0.70794677734375, 0.70111083984375, 0.72064208984375, 0.70587158203125, 0.71868896484375, 0.70806884765625, 0.70574951171875, 0.68267822265625, 0.70697021484375, 0.69793701171875, 0.66278076171875, 0.69158935546875, 0.67816162109375, 0.69622802734375, 0.72137451171875, 0.73223876953125, 0.70843505859375, 0.70208740234375, 0.70684814453125, 0.68963623046875, 0.67681884765625, 0.70941162109375, 0.70001220703125, 0.67584228515625, 0.70623779296875, 0.69476318359375, 0.65411376953125, 0.65606689453125, 0.68572998046875, 0.68548583984375, 0.71881103515625, 0.69683837890625, 0.69488525390625, 0.70135498046875, 0.68121337890625, 0.71368408203125, 0.70098876953125, 0.66448974609375, 0.69659423828125, 0.66595458984375, 0.67901611328125, 0.68963623046875, 0.70770263671875, 0.71929931640625, 0.70867919921875, 0.70880126953125, 0.70074462890625, 0.69659423828125, 0.69610595703125, 0.68450927734375, 0.68585205078125, 0.69805908203125, 0.68780517578125, 0.66241455078125, 0.67108154296875, 0.70733642578125, 0.66363525390625, 0.67193603515625, 0.65606689453125, 0.65875244140625, 0.69390869140625, 0.70062255859375, 0.68475341796875, 0.68731689453125, 0.70428466796875, 0.70159912109375, 0.67498779296875, 0.67669677734375, 0.67791748046875, 0.69622802734375, 0.73956298828125, 0.70831298828125, 0.69110107421875, 0.68731689453125, 0.69940185546875, 0.68939208984375, 0.72625732421875, 0.68572998046875, 0.70013427734375, 0.67034912109375, 0.69012451171875, 0.66912841796875, 0.71429443359375, 0.71002197265625, 0.68878173828125, 0.70513916015625, 0.70416259765625, 0.72637939453125, 0.68536376953125, 0.72344970703125, 0.70367431640625, 0.69354248046875, 0.69293212890625, 0.68231201171875, 0.70648193359375, 0.66375732421875, 0.69427490234375, 0.69927978515625, 0.69512939453125, 0.70269775390625, 0.67315673828125, 0.69952392578125, 0.66949462890625, 0.67950439453125, 0.68157958984375, 0.70916748046875, 0.71893310546875, 0.68292236328125, 0.69525146484375, 0.69610595703125, 0.66986083984375, 0.67803955078125, 0.68170166015625, 0.65045166015625, 0.73089599609375, 0.67095947265625, 0.68035888671875, 0.69488525390625, 0.69793701171875, 0.71917724609375, 0.67120361328125, 0.69256591796875, 0.68841552734375, 0.69500732421875, 0.69281005859375, 0.69635009765625, 0.67840576171875, 0.66607666015625, 0.68060302734375, 0.66693115234375, 0.66265869140625, 0.67803955078125, 0.69061279296875, 0.67901611328125, 0.68890380859375, 0.70489501953125, 0.70269775390625, 0.69561767578125, 0.67864990234375, 0.63519287109375, 0.67132568359375, 0.69891357421875, 0.68511962890625, 0.66571044921875, 0.70538330078125, 0.67083740234375, 0.68975830078125, 0.68377685546875, 0.68365478515625, 0.70172119140625, 0.70428466796875, 0.66571044921875, 0.72711181640625, 0.69561767578125, 0.68011474609375, 0.69573974609375, 0.71832275390625, 0.68218994140625, 0.70538330078125, 0.69061279296875, 0.70306396484375, 0.68157958984375, 0.67694091796875, 0.70379638671875, 0.70843505859375, 0.67388916015625, 0.68585205078125, 0.67108154296875, 0.68121337890625, 0.66632080078125, 0.71246337890625, 0.71319580078125, 0.65228271484375, 0.67547607421875, 0.66656494140625, 0.67437744140625, 0.67462158203125, 0.68389892578125, 0.67523193359375, 0.67987060546875, 0.68023681640625, 0.68231201171875, 0.66912841796875, 0.67584228515625, 0.65777587890625, 0.65411376953125, 0.69134521484375, 0.64666748046875, 0.67108154296875, 0.65997314453125, 0.69110107421875, 0.65509033203125, 0.69818115234375, 0.67498779296875, 0.68096923828125, 0.71612548828125, 0.68170166015625, 0.68902587890625, 0.70953369140625, 0.69598388671875, 0.69219970703125, 0.66949462890625, 0.70806884765625, 0.66485595703125, 0.67364501953125, 0.66680908203125, 0.64178466796875, 0.68414306640625, 0.66973876953125, 0.70501708984375, 0.69097900390625, 0.68817138671875, 0.67852783203125, 0.70916748046875, 0.67987060546875, 0.69537353515625, 0.69915771484375, 0.69488525390625, 0.70562744140625, 0.66021728515625, 0.67718505859375, 0.67742919921875, 0.72222900390625, 0.70147705078125, 0.70599365234375, 0.70281982421875, 0.70745849609375, 0.68609619140625, 0.71270751953125, 0.67254638671875, 0.70013427734375, 0.67181396484375, 0.69989013671875, 0.69818115234375, 0.71612548828125, 0.70025634765625, 0.69500732421875, 0.68707275390625, 0.68121337890625, 0.66241455078125, 0.69769287109375, 0.69744873046875, 0.69732666015625, 0.69036865234375, 0.69036865234375, 0.68328857421875, 0.68316650390625, 0.70452880859375, 0.66156005859375, 0.69622802734375, 0.68682861328125, 0.68731689453125, 0.69622802734375, 0.69976806640625, 0.71417236328125, 0.69708251953125, 0.69000244140625, 0.69500732421875, 0.68206787109375, 0.70526123046875, 0.71612548828125, 0.65277099609375, 0.69232177734375, 0.67535400390625, 0.64324951171875, 0.69427490234375, 0.67059326171875, 0.66094970703125, 0.66693115234375, 0.69647216796875, 0.68548583984375, 0.71026611328125, 0.69427490234375, 0.66375732421875, 0.68182373046875, 0.70037841796875, 0.67706298828125, 0.72137451171875, 0.71563720703125, 0.69073486328125, 0.71466064453125, 0.67816162109375, 0.70587158203125, 0.70758056640625, 0.68572998046875, 0.70843505859375, 0.71160888671875, 0.69427490234375, 0.73651123046875, 0.68365478515625, 0.68829345703125, 0.67388916015625, 0.73321533203125, 0.67633056640625, 0.69744873046875, 0.69403076171875, 0.71002197265625, 0.68988037109375, 0.68511962890625, 0.67974853515625, 0.68341064453125, 0.69976806640625, 0.69781494140625, 0.70562744140625, 0.71429443359375, 0.70501708984375, 0.67510986328125, 0.74542236328125, 0.69744873046875, 0.69305419921875, 0.69342041015625, 0.71026611328125, 0.65496826171875, 0.66827392578125, 0.70318603515625, 0.68670654296875, 0.69281005859375, 0.69207763671875, 0.69573974609375, 0.70892333984375, 0.65716552734375, 0.68609619140625, 0.68609619140625, 0.65167236328125, 0.69281005859375, 0.68218994140625, 0.70220947265625, 0.68548583984375, 0.69207763671875, 0.69757080078125, 0.68499755859375, 0.68572998046875, 0.69427490234375, 0.71051025390625, 0.70208740234375, 0.69879150390625, 0.70562744140625, 0.72589111328125, 0.70294189453125, 0.69415283203125, 0.72027587890625, 0.70697021484375, 0.68267822265625, 0.68548583984375, 0.68157958984375, 0.68145751953125, 0.66973876953125, 0.66864013671875, 0.68621826171875, 0.66815185546875, 0.68853759765625, 0.69122314453125, 0.70062255859375, 0.69439697265625, 0.69549560546875, 0.68963623046875, 0.68731689453125, 0.67999267578125, 0.69720458984375, 0.68743896484375, 0.71380615234375, 0.69158935546875, 0.69903564453125, 0.71282958984375, 0.71795654296875, 0.70562744140625, 0.69268798828125, 0.66241455078125, 0.70513916015625, 0.68194580078125, 0.70025634765625, 0.69451904296875, 0.67498779296875, 0.66827392578125, 0.69268798828125, 0.66705322265625, 0.69781494140625, 0.67474365234375, 0.71197509765625, 0.66534423828125, 0.64666748046875, 0.69097900390625, 0.64105224609375, 0.66949462890625, 0.71466064453125, 0.65863037109375, 0.67559814453125, 0.64544677734375, 0.69696044921875, 0.67987060546875, 0.71282958984375, 0.66864013671875, 0.68109130859375, 0.67913818359375, 0.66485595703125, 0.70318603515625, 0.67755126953125, 0.68365478515625, 0.67620849609375, 0.68402099609375, 0.65887451171875, 0.68353271484375, 0.67095947265625, 0.66949462890625, 0.68792724609375, 0.67645263671875, 0.67730712890625, 0.67291259765625, 0.68048095703125, 0.68682861328125, 0.69793701171875, 0.69927978515625, 0.66253662109375, 0.68853759765625, 0.69329833984375, 0.68634033203125, 0.66656494140625, 0.68939208984375, 0.67803955078125, 0.68756103515625, 0.69500732421875, 0.70867919921875, 0.69317626953125, 0.70428466796875, 0.71600341796875, 0.68853759765625, 0.69073486328125, 0.68731689453125, 0.65411376953125, 0.66839599609375, 0.66448974609375, 0.67584228515625, 0.66326904296875, 0.68756103515625, 0.69415283203125, 0.68975830078125, 0.68914794921875, 0.68341064453125, 0.68109130859375, 0.71734619140625, 0.68646240234375, 0.67706298828125, 0.70538330078125, 0.69427490234375, 0.69036865234375, 0.69854736328125, 0.68670654296875, 0.70721435546875, 0.71087646484375, 0.70074462890625, 0.68109130859375, 0.69647216796875, 0.70416259765625, 0.68450927734375, 0.67364501953125, 0.68988037109375, 0.64483642578125, 0.70135498046875, 0.65740966796875, 0.70111083984375, 0.70526123046875, 0.67279052734375, 0.66644287109375, 0.69122314453125, 0.67730712890625, 0.70648193359375, 0.64459228515625, 0.67742919921875, 0.69793701171875, 0.70233154296875, 0.70343017578125, 0.68414306640625, 0.66241455078125, 0.68731689453125, 0.66595458984375, 0.66741943359375, 0.67340087890625, 0.70013427734375, 0.67840576171875, 0.70404052734375, 0.69744873046875, 0.70404052734375, 0.68817138671875, 0.68328857421875, 0.69635009765625, 0.70159912109375, 0.68463134765625, 0.69537353515625, 0.69500732421875, 0.67474365234375, 0.68341064453125, 0.69097900390625, 0.69024658203125, 0.68389892578125, 0.70526123046875, 0.69146728515625, 0.70111083984375, 0.67987060546875, 0.68365478515625, 0.69586181640625, 0.66058349609375, 0.68682861328125, 0.67730712890625, 0.71844482421875, 0.68572998046875, 0.67681884765625, 0.68975830078125, 0.67938232421875, 0.65753173828125, 0.71405029296875, 0.68316650390625, 0.69622802734375, 0.67962646484375, 0.68927001953125, 0.68585205078125, 0.68304443359375, 0.69598388671875, 0.70233154296875, 0.71307373046875, 0.69000244140625, 0.70782470703125, 0.69537353515625, 0.67779541015625, 0.67767333984375, 0.70697021484375, 0.72100830078125, 0.68865966796875, 0.69940185546875, 0.68756103515625, 0.69464111328125, 0.70452880859375, 0.69476318359375, 0.70635986328125, 0.68255615234375, 0.67877197265625, 0.68609619140625, 0.67706298828125, 0.67938232421875, 0.68231201171875, 0.69256591796875, 0.67523193359375, 0.68609619140625, 0.66705322265625, 0.69195556640625, 0.68707275390625, 0.70831298828125, 0.66619873046875, 0.66265869140625, 0.70306396484375, 0.69488525390625, 0.70660400390625, 0.67315673828125, 0.68206787109375, 0.65386962890625, 0.69561767578125, 0.69976806640625, 0.67303466796875, 0.66925048828125, 0.69500732421875, 0.68402099609375, 0.71380615234375, 0.68353271484375, 0.72113037109375, 0.68963623046875, 0.70245361328125, 0.67498779296875, 0.66961669921875, 0.69793701171875, 0.68951416015625, 0.70880126953125, 0.71539306640625, 0.69281005859375, 0.70745849609375, 0.71099853515625, 0.70330810546875, 0.72015380859375, 0.69610595703125, 0.68475341796875, 0.66937255859375, 0.68048095703125, 0.68560791015625, 0.67584228515625, 0.69903564453125, 0.71063232421875, 0.70159912109375, 0.73175048828125, 0.69854736328125, 0.70172119140625, 0.68975830078125, 0.68072509765625, 0.70867919921875, 0.69024658203125, 0.71234130859375, 0.69476318359375, 0.69964599609375, 0.71234130859375, 0.70025634765625, 0.68304443359375, 0.71490478515625, 0.69061279296875, 0.69903564453125, 0.69317626953125, 0.67938232421875, 0.67816162109375, 0.70428466796875, 0.69940185546875, 0.69793701171875, 0.67193603515625, 0.69085693359375, 0.65753173828125, 0.68731689453125, 0.66436767578125, 0.68536376953125, 0.67022705078125, 0.69366455078125, 0.67156982421875, 0.68109130859375, 0.70208740234375, 0.70819091796875, 0.69036865234375, 0.68560791015625, 0.70330810546875, 0.69696044921875, 0.69427490234375, 0.67950439453125, 0.67230224609375, 0.66400146484375, 0.69427490234375, 0.69830322265625, 0.67340087890625, 0.69586181640625, 0.69097900390625, 0.69537353515625, 0.68646240234375, 0.67877197265625, 0.69378662109375, 0.68621826171875, 0.70611572265625, 0.66864013671875, 0.69818115234375, 0.66949462890625, 0.68304443359375, 0.70062255859375, 0.70672607421875, 0.69415283203125, 0.72271728515625, 0.68255615234375, 0.69696044921875, 0.66656494140625, 0.69488525390625, 0.72283935546875, 0.68975830078125, 0.70135498046875, 0.71282958984375, 0.67974853515625, 0.72772216796875, 0.68511962890625, 0.67987060546875, 0.69110107421875, 0.69647216796875, 0.67974853515625, 0.69390869140625, 0.68914794921875, 0.68853759765625, 0.69293212890625, 0.73077392578125, 0.67547607421875, 0.69317626953125, 0.70758056640625, 0.69097900390625, 0.69451904296875, 0.69842529296875, 0.68634033203125, 0.65252685546875, 0.70428466796875, 0.68841552734375, 0.67889404296875, 0.69610595703125, 0.69171142578125, 0.67694091796875, 0.68316650390625, 0.69671630859375, 0.69964599609375, 0.69476318359375, 0.72869873046875, 0.67645263671875, 0.70452880859375, 0.71307373046875, 0.69451904296875, 0.70001220703125, 0.67144775390625, 0.68536376953125, 0.68963623046875, 0.69378662109375, 0.69525146484375, 0.67779541015625, 0.69000244140625, 0.69219970703125, 0.65484619140625, 0.68768310546875, 0.73687744140625, 0.69415283203125, 0.71234130859375, 0.67730712890625, 0.66961669921875, 0.69744873046875, 0.69903564453125, 0.67950439453125, 0.68096923828125, 0.69122314453125, 0.68182373046875, 0.67340087890625, 0.68035888671875, 0.67718505859375, 0.67364501953125, 0.68548583984375, 0.68316650390625, 0.71270751953125, 0.67303466796875, 0.70843505859375, 0.67864990234375, 0.69708251953125, 0.69207763671875, 0.68499755859375, 0.72113037109375, 0.67926025390625, 0.69476318359375, 0.67657470703125, 0.67669677734375, 0.69403076171875, 0.68121337890625, 0.68951416015625, 0.69720458984375, 0.69000244140625, 0.68035888671875, 0.68988037109375, 0.72125244140625, 0.69158935546875, 0.70184326171875, 0.66632080078125, 0.67242431640625, 0.66876220703125, 0.71002197265625, 0.67413330078125, 0.67633056640625, 0.70806884765625, 0.65618896484375, 0.69659423828125, 0.68609619140625, 0.69464111328125, 0.69134521484375, 0.67926025390625, 0.69805908203125, 0.70159912109375, 0.68231201171875, 0.68121337890625, 0.68511962890625, 0.70294189453125, 0.69305419921875, 0.68890380859375, 0.68768310546875, 0.69903564453125, 0.67486572265625, 0.67767333984375, 0.70880126953125, 0.66973876953125, 0.69293212890625, 0.69647216796875, 0.67974853515625, 0.68768310546875, 0.67327880859375, 0.69671630859375, 0.67315673828125, 0.69403076171875, 0.71856689453125, 0.69488525390625, 0.74395751953125, 0.70672607421875, 0.70648193359375, 0.70062255859375, 0.70623779296875, 0.68133544921875, 0.68011474609375, 0.67547607421875, 0.67132568359375, 0.68829345703125, 0.69659423828125, 0.70184326171875, 0.70318603515625, 0.70098876953125, 0.69683837890625, 0.69561767578125, 0.67083740234375, 0.69976806640625, 0.71759033203125, 0.69622802734375, 0.68548583984375, 0.70513916015625, 0.70172119140625, 0.68206787109375, 0.68389892578125, 0.69940185546875, 0.70123291015625, 0.69012451171875, 0.67266845703125, 0.70867919921875, 0.71148681640625, 0.71148681640625, 0.70318603515625, 0.69964599609375, 0.70428466796875, 0.72027587890625, 0.72894287109375, 0.68072509765625, 0.71014404296875, 0.68060302734375, 0.69903564453125, 0.67950439453125, 0.71307373046875, 0.68878173828125, 0.68304443359375, 0.68463134765625, 0.69525146484375, 0.69598388671875, 0.69110107421875, 0.70513916015625, 0.69854736328125, 0.67315673828125, 0.71014404296875, 0.67608642578125, 0.67095947265625, 0.68414306640625, 0.66168212890625, 0.67303466796875, 0.67742919921875, 0.67950439453125, 0.68060302734375, 0.67059326171875, 0.68035888671875, 0.66448974609375, 0.69183349609375, 0.67449951171875, 0.70599365234375, 0.67425537109375, 0.67706298828125, 0.64630126953125, 0.67303466796875, 0.67547607421875, 0.67120361328125, 0.68572998046875, 0.70074462890625, 0.67388916015625, 0.69622802734375, 0.65570068359375, 0.68829345703125, 0.70330810546875, 0.69940185546875, 0.69293212890625, 0.73065185546875, 0.69110107421875, 0.68304443359375, 0.69403076171875, 0.70953369140625, 0.70794677734375, 0.69927978515625, 0.70416259765625, 0.68963623046875, 0.66265869140625, 0.68621826171875, 0.68023681640625, 0.68109130859375, 0.67083740234375, 0.69671630859375, 0.68157958984375, 0.69000244140625, 0.67474365234375, 0.69805908203125, 0.70489501953125, 0.67852783203125, 0.67083740234375, 0.66168212890625, 0.70819091796875, 0.68756103515625, 0.69696044921875, 0.67425537109375, 0.67266845703125, 0.69696044921875, 0.68035888671875, 0.72003173828125, 0.69805908203125, 0.67620849609375, 0.67999267578125, 0.71710205078125, 0.69635009765625, 0.65863037109375, 0.71307373046875, 0.68499755859375, 0.67901611328125, 0.68060302734375, 0.67022705078125, 0.68060302734375, 0.66436767578125, 0.67681884765625, 0.69012451171875, 0.67449951171875, 0.67401123046875, 0.68121337890625, 0.70867919921875, 0.66180419921875, 0.65606689453125, 0.65716552734375, 0.67620849609375, 0.68597412109375, 0.67608642578125, 0.68182373046875, 0.70379638671875, 0.68414306640625, 0.69842529296875, 0.66973876953125, 0.69061279296875, 0.68963623046875, 0.70367431640625, 0.69097900390625, 0.68475341796875, 0.68072509765625, 0.70135498046875, 0.67254638671875, 0.69000244140625, 0.68255615234375, 0.67608642578125, 0.70123291015625, 0.68682861328125, 0.66778564453125, 0.67462158203125, 0.70025634765625, 0.70257568359375, 0.66131591796875, 0.68170166015625, 0.68316650390625, 0.69647216796875, 0.69537353515625, 0.70574951171875, 0.69097900390625, 0.68695068359375, 0.72991943359375, 0.68670654296875, 0.69146728515625, 0.69818115234375, 0.66705322265625, 0.66424560546875, 0.68707275390625, 0.67657470703125, 0.66827392578125, 0.66131591796875, 0.66778564453125, 0.69610595703125, 0.71258544921875, 0.69122314453125, 0.69891357421875, 0.65423583984375, 0.68194580078125, 0.67218017578125, 0.65142822265625, 0.64068603515625, 0.70770263671875, 0.68829345703125, 0.67596435546875, 0.69110107421875, 0.66851806640625, 0.72015380859375, 0.66973876953125, 0.71514892578125, 0.68328857421875, 0.67120361328125, 0.68524169921875, 0.67645263671875, 0.67510986328125, 0.67071533203125, 0.69818115234375, 0.67950439453125, 0.69732666015625, 0.69219970703125, 0.66961669921875, 0.65350341796875, 0.67047119140625, 0.67095947265625, 0.68731689453125, 0.68658447265625, 0.67022705078125, 0.69573974609375, 0.70477294921875, 0.67926025390625, 0.68707275390625, 0.66876220703125, 0.70379638671875, 0.67620849609375, 0.69403076171875, 0.70135498046875, 0.67193603515625, 0.68792724609375, 0.67205810546875, 0.69537353515625, 0.72235107421875, 0.68084716796875, 0.69049072265625, 0.68670654296875, 0.71673583984375, 0.69439697265625, 0.68695068359375, 0.68731689453125, 0.65496826171875, 0.70440673828125, 0.68011474609375, 0.69439697265625, 0.70391845703125, 0.68743896484375, 0.69366455078125, 0.67926025390625, 0.71771240234375, 0.68536376953125, 0.70172119140625, 0.66302490234375, 0.70709228515625, 0.69561767578125, 0.70404052734375, 0.71392822265625, 0.72125244140625, 0.71197509765625, 0.70025634765625, 0.67095947265625, 0.70672607421875, 0.67926025390625, 0.65924072265625, 0.69610595703125, 0.67181396484375, 0.68743896484375, 0.67230224609375, 0.68341064453125, 0.69464111328125, 0.66131591796875, 0.69390869140625, 0.68902587890625, 0.70465087890625, 0.69586181640625, 0.68829345703125, 0.67828369140625, 0.66424560546875, 0.69891357421875, 0.67047119140625, 0.69354248046875, 0.67816162109375, 0.68328857421875, 0.67486572265625, 0.67303466796875, 0.68438720703125, 0.66534423828125, 0.69720458984375, 0.68243408203125, 0.68682861328125, 0.67327880859375, 0.68267822265625, 0.69879150390625, 0.67486572265625, 0.70867919921875, 0.67901611328125, 0.69866943359375, 0.66265869140625, 0.68060302734375, 0.67413330078125, 0.68035888671875, 0.70660400390625, 0.69097900390625, 0.67974853515625, 0.67718505859375, 0.68145751953125, 0.67987060546875, 0.70123291015625, 0.68756103515625, 0.70355224609375, 0.70147705078125, 0.71026611328125, 0.68280029296875, 0.68206787109375, 0.69110107421875, 0.68621826171875, 0.67938232421875, 0.67657470703125, 0.68267822265625, 0.69854736328125, 0.68402099609375, 0.69818115234375, 0.68023681640625, 0.70379638671875, 0.72259521484375, 0.73468017578125, 0.68707275390625, 0.72296142578125, 0.72174072265625, 0.67779541015625, 0.68792724609375, 0.68060302734375, 0.67132568359375, 0.69525146484375, 0.66339111328125, 0.69805908203125, 0.68243408203125, 0.70086669921875, 0.66815185546875, 0.70965576171875, 0.68048095703125, 0.68304443359375, 0.68548583984375, 0.69219970703125, 0.67181396484375, 0.67474365234375, 0.68524169921875, 0.70306396484375, 0.71685791015625, 0.69036865234375, 0.73187255859375, 0.68695068359375, 0.66412353515625, 0.66949462890625, 0.68328857421875, 0.66241455078125, 0.68182373046875, 0.68780517578125, 0.68951416015625, 0.69989013671875, 0.66400146484375, 0.69317626953125, 0.69476318359375, 0.69586181640625, 0.66033935546875, 0.66534423828125, 0.68682861328125, 0.69818115234375, 0.68597412109375, 0.68450927734375, 0.66619873046875, 0.70306396484375, 0.69573974609375, 0.67706298828125, 0.66986083984375, 0.70867919921875, 0.67950439453125, 0.69366455078125, 0.67266845703125, 0.71527099609375, 0.69915771484375, 0.69744873046875, 0.69268798828125, 0.70489501953125, 0.68463134765625, 0.69378662109375, 0.69854736328125, 0.68402099609375, 0.68121337890625, 0.69927978515625, 0.66412353515625, 0.69854736328125, 0.70367431640625, 0.70806884765625, 0.72454833984375, 0.70574951171875, 0.69158935546875, 0.69293212890625, 0.66851806640625, 0.69525146484375, 0.68939208984375, 0.64300537109375, 0.70343017578125, 0.67376708984375, 0.67230224609375, 0.67999267578125, 0.68170166015625, 0.69635009765625, 0.71759033203125, 0.68548583984375, 0.71685791015625, 0.69134521484375, 0.65423583984375, 0.67218017578125, 0.68121337890625, 0.67877197265625, 0.69696044921875, 0.68243408203125, 0.69049072265625, 0.69000244140625, 0.64202880859375, 0.69696044921875, 0.66192626953125, 0.68646240234375, 0.68011474609375, 0.67657470703125, 0.68499755859375, 0.68560791015625, 0.67425537109375, 0.67218017578125, 0.69683837890625, 0.66302490234375, 0.67864990234375, 0.68267822265625, 0.67913818359375, 0.65777587890625, 0.66741943359375, 0.69464111328125, 0.69219970703125, 0.70440673828125, 0.70843505859375, 0.70062255859375, 0.68084716796875, 0.69964599609375, 0.68914794921875, 0.65118408203125, 0.68792724609375, 0.68841552734375, 0.67962646484375, 0.73931884765625, 0.69378662109375, 0.72320556640625, 0.65887451171875, 0.71893310546875, 0.68829345703125, 0.68841552734375, 0.68145751953125, 0.68890380859375, 0.71063232421875, 0.66986083984375, 0.69879150390625, 0.71112060546875, 0.69427490234375, 0.71185302734375, 0.69024658203125, 0.71392822265625, 0.69757080078125, 0.66912841796875, 0.68414306640625, 0.71270751953125, 0.67376708984375, 0.68450927734375, 0.69549560546875, 0.70953369140625, 0.67681884765625, 0.69610595703125, 0.67742919921875, 0.69073486328125, 0.70672607421875, 0.72113037109375, 0.68914794921875, 0.67926025390625, 0.69476318359375, 0.67291259765625, 0.68292236328125, 0.68719482421875, 0.67779541015625, 0.67645263671875, 0.68524169921875, 0.67828369140625, 0.67828369140625, 0.66912841796875, 0.69586181640625, 0.67291259765625, 0.67864990234375, 0.69305419921875, 0.67108154296875, 0.66156005859375, 0.68035888671875, 0.66448974609375, 0.71551513671875, 0.68072509765625, 0.70281982421875, 0.67230224609375, 0.67572021484375, 0.68145751953125, 0.65887451171875, 0.69793701171875, 0.66119384765625, 0.67840576171875, 0.68939208984375, 0.69024658203125, 0.70404052734375, 0.70526123046875, 0.67303466796875, 0.68084716796875, 0.69586181640625, 0.67742919921875, 0.67645263671875, 0.68377685546875, 0.65948486328125, 0.67144775390625, 0.68243408203125, 0.70050048828125, 0.69476318359375, 0.71221923828125, 0.66607666015625, 0.68292236328125, 0.71710205078125, 0.70587158203125, 0.70989990234375, 0.68621826171875, 0.68939208984375, 0.68255615234375, 0.69097900390625, 0.70062255859375, 0.70257568359375, 0.69464111328125, 0.69219970703125, 0.66937255859375, 0.67926025390625, 0.68511962890625, 0.66473388671875, 0.69903564453125, 0.66876220703125, 0.66119384765625, 0.70037841796875, 0.68658447265625, 0.69049072265625, 0.69732666015625, 0.68548583984375, 0.67999267578125, 0.68585205078125, 0.67938232421875, 0.69268798828125, 0.70135498046875, 0.68426513671875, 0.69586181640625, 0.68109130859375, 0.69549560546875, 0.67987060546875, 0.69732666015625, 0.68035888671875, 0.67303466796875, 0.64447021484375, 0.67413330078125, 0.66412353515625, 0.70501708984375, 0.64727783203125, 0.67572021484375, 0.69049072265625, 0.68475341796875, 0.68402099609375, 0.67083740234375, 0.67974853515625, 0.65045166015625, 0.68243408203125, 0.68829345703125, 0.67034912109375, 0.69805908203125, 0.70538330078125, 0.67864990234375, 0.68890380859375, 0.67352294921875, 0.69696044921875, 0.67413330078125, 0.70538330078125, 0.67034912109375, 0.69830322265625, 0.67120361328125, 0.67742919921875, 0.67657470703125, 0.66265869140625, 0.69586181640625, 0.68719482421875, 0.68780517578125, 0.68011474609375, 0.67462158203125, 0.66326904296875, 0.67608642578125, 0.70245361328125, 0.70013427734375, 0.69573974609375, 0.68414306640625, 0.66986083984375, 0.67840576171875, 0.70465087890625, 0.69378662109375, 0.69610595703125, 0.68536376953125, 0.68902587890625, 0.68377685546875, 0.69781494140625, 0.71636962890625, 0.68902587890625, 0.69610595703125, 0.69940185546875, 0.70123291015625, 0.69732666015625, 0.68084716796875, 0.71014404296875, 0.67523193359375, 0.69024658203125, 0.67047119140625, 0.68804931640625, 0.66131591796875, 0.66558837890625, 0.69390869140625, 0.68206787109375, 0.66925048828125, 0.69439697265625, 0.66729736328125, 0.68341064453125, 0.67913818359375, 0.68804931640625, 0.68829345703125, 0.68646240234375, 0.69451904296875, 0.67303466796875, 0.69952392578125, 0.69964599609375, 0.69036865234375, 0.66644287109375, 0.66217041015625, 0.68243408203125, 0.67584228515625, 0.70037841796875, 0.67535400390625, 0.69451904296875, 0.68768310546875, 0.67828369140625, 0.68145751953125, 0.69110107421875, 0.67620849609375, 0.66241455078125, 0.71124267578125, 0.67535400390625, 0.67596435546875, 0.69451904296875, 0.69329833984375, 0.69708251953125, 0.70904541015625, 0.67803955078125, 0.70770263671875, 0.68475341796875, 0.69866943359375, 0.70123291015625, 0.70416259765625, 0.70062255859375, 0.70697021484375, 0.70623779296875, 0.69146728515625, 0.67620849609375, 0.71868896484375, 0.68231201171875, 0.67889404296875, 0.71697998046875, 0.68341064453125, 0.69879150390625, 0.69085693359375, 0.69171142578125, 0.68243408203125, 0.67803955078125, 0.72723388671875, 0.71563720703125, 0.68084716796875, 0.68853759765625, 0.73553466796875, 0.70709228515625, 0.73358154296875, 0.67449951171875, 0.69403076171875, 0.65887451171875, 0.71929931640625, 0.69854736328125, 0.70062255859375, 0.67254638671875, 0.67742919921875, 0.70574951171875, 0.68218994140625, 0.70184326171875, 0.69842529296875, 0.70806884765625, 0.65594482421875, 0.66351318359375, 0.70220947265625, 0.68804931640625, 0.69036865234375, 0.68768310546875, 0.67974853515625, 0.69085693359375, 0.66302490234375, 0.68060302734375, 0.67645263671875, 0.70025634765625, 0.67864990234375, 0.66778564453125, 0.67681884765625, 0.69537353515625, 0.68109130859375, 0.67669677734375, 0.71441650390625, 0.70123291015625, 0.69964599609375, 0.68048095703125, 0.68609619140625, 0.68548583984375, 0.67254638671875, 0.70330810546875, 0.66741943359375, 0.70745849609375, 0.71380615234375, 0.67523193359375, 0.68780517578125, 0.68817138671875, 0.68328857421875, 0.66656494140625, 0.67242431640625, 0.69342041015625, 0.69720458984375, 0.71087646484375, 0.68853759765625, 0.71295166015625, 0.68621826171875, 0.67987060546875, 0.72137451171875, 0.68646240234375, 0.68841552734375, 0.69268798828125, 0.68695068359375, 0.69683837890625, 0.71124267578125, 0.70428466796875, 0.70989990234375, 0.71343994140625, 0.70867919921875, 0.71148681640625, 0.70172119140625, 0.69500732421875, 0.68670654296875, 0.69879150390625, 0.71002197265625, 0.67352294921875, 0.69232177734375, 0.69671630859375, 0.70159912109375, 0.67742919921875, 0.68829345703125, 0.66790771484375, 0.69561767578125, 0.68035888671875, 0.66107177734375, 0.67303466796875, 0.66949462890625, 0.66876220703125, 0.70379638671875, 0.67205810546875, 0.69537353515625, 0.67620849609375, 0.69610595703125, 0.67510986328125, 0.68206787109375, 0.68487548828125, 0.67156982421875, 0.66571044921875, 0.68487548828125, 0.67095947265625, 0.66632080078125, 0.69635009765625, 0.66375732421875, 0.70440673828125, 0.70416259765625, 0.69915771484375, 0.67181396484375, 0.66998291015625, 0.67755126953125, 0.68511962890625, 0.64801025390625, 0.69403076171875, 0.67181396484375, 0.69647216796875, 0.68585205078125, 0.69976806640625, 0.69793701171875, 0.67779541015625, 0.67767333984375, 0.71649169921875, 0.67669677734375, 0.68792724609375, 0.67816162109375, 0.67144775390625, 0.67340087890625, 0.70184326171875, 0.70037841796875, 0.70989990234375, 0.67755126953125, 0.70001220703125, 0.69354248046875, 0.70404052734375, 0.69427490234375, 0.68829345703125, 0.69207763671875, 0.71038818359375, 0.68011474609375, 0.70050048828125, 0.69256591796875, 0.69232177734375, 0.64959716796875, 0.69403076171875, 0.69989013671875, 0.66094970703125, 0.69647216796875, 0.67730712890625, 0.69415283203125, 0.68902587890625, 0.68707275390625, 0.69403076171875, 0.70050048828125, 0.69354248046875, 0.69732666015625, 0.69305419921875, 0.66339111328125, 0.70196533203125, 0.66387939453125, 0.69696044921875, 0.68951416015625, 0.67144775390625, 0.68585205078125, 0.69635009765625, 0.67547607421875, 0.67230224609375, 0.65985107421875, 0.71209716796875, 0.67926025390625, 0.68023681640625, 0.66058349609375, 0.65130615234375, 0.69244384765625, 0.68780517578125, 0.68341064453125, 0.69525146484375, 0.68182373046875, 0.66802978515625, 0.70013427734375, 0.69549560546875, 0.67926025390625, 0.69036865234375, 0.69793701171875, 0.69866943359375, 0.70843505859375, 0.70391845703125, 0.67523193359375, 0.67718505859375, 0.70623779296875, 0.68780517578125, 0.67498779296875, 0.70843505859375, 0.70269775390625, 0.69232177734375, 0.72894287109375, 0.70135498046875, 0.70062255859375, 0.73040771484375, 0.70465087890625, 0.69219970703125, 0.71453857421875, 0.70172119140625, 0.68743896484375, 0.68182373046875, 0.70794677734375, 0.68780517578125, 0.71026611328125, 0.67999267578125, 0.69793701171875, 0.70208740234375, 0.71343994140625, 0.69390869140625, 0.67596435546875, 0.67694091796875, 0.67657470703125, 0.68853759765625, 0.72857666015625, 0.69793701171875, 0.67657470703125, 0.69793701171875, 0.68292236328125, 0.72747802734375, 0.69720458984375, 0.70196533203125, 0.73272705078125, 0.68719482421875, 0.69866943359375, 0.67974853515625, 0.71600341796875, 0.67315673828125, 0.67987060546875, 0.69781494140625, 0.68475341796875, 0.66094970703125, 0.71856689453125, 0.69293212890625, 0.67938232421875, 0.65472412109375, 0.67535400390625, 0.69012451171875, 0.69927978515625, 0.70916748046875, 0.67987060546875, 0.68243408203125, 0.70587158203125, 0.70086669921875, 0.65985107421875, 0.66888427734375, 0.65216064453125, 0.67071533203125, 0.65484619140625, 0.66741943359375, 0.70611572265625, 0.68829345703125, 0.71319580078125, 0.68646240234375, 0.69366455078125, 0.66302490234375, 0.67584228515625, 0.68878173828125, 0.70220947265625, 0.70953369140625, 0.66571044921875, 0.67022705078125, 0.69305419921875, 0.68634033203125, 0.70257568359375, 0.69232177734375, 0.66571044921875, 0.71514892578125, 0.68280029296875, 0.70904541015625, 0.67950439453125, 0.69964599609375, 0.66693115234375, 0.69476318359375, 0.69378662109375, 0.71466064453125, 0.71185302734375, 0.68341064453125, 0.69085693359375, 0.68853759765625, 0.69024658203125, 0.69940185546875, 0.69830322265625, 0.69757080078125, 0.67401123046875, 0.68121337890625, 0.70013427734375, 0.70025634765625, 0.69903564453125, 0.69586181640625, 0.70550537109375, 0.67913818359375, 0.64825439453125, 0.65130615234375, 0.69903564453125, 0.65179443359375, 0.67230224609375, 0.69952392578125, 0.68829345703125, 0.70098876953125, 0.69610595703125, 0.71197509765625, 0.70550537109375, 0.69769287109375, 0.66339111328125, 0.68963623046875, 0.69232177734375, 0.69415283203125, 0.70782470703125, 0.68353271484375, 0.71380615234375, 0.68804931640625, 0.70233154296875, 0.69635009765625, 0.66058349609375, 0.68499755859375, 0.68438720703125, 0.67291259765625, 0.65350341796875, 0.68475341796875, 0.69000244140625, 0.69769287109375, 0.68682861328125, 0.69085693359375, 0.67059326171875, 0.69964599609375, 0.69903564453125, 0.64923095703125, 0.67572021484375, 0.68841552734375, 0.66461181640625, 0.67803955078125, 0.69036865234375, 0.70928955078125, 0.67999267578125, 0.72418212890625, 0.68988037109375, 0.70489501953125, 0.69305419921875, 0.68328857421875, 0.71343994140625, 0.67877197265625, 0.70538330078125, 0.67669677734375, 0.71356201171875, 0.67840576171875, 0.70562744140625, 0.69964599609375, 0.68536376953125, 0.70806884765625, 0.66558837890625, 0.67938232421875, 0.70733642578125, 0.70989990234375, 0.66522216796875, 0.68670654296875, 0.66107177734375, 0.71759033203125, 0.69207763671875, 0.68548583984375, 0.68658447265625, 0.70587158203125, 0.68743896484375, 0.69976806640625, 0.69549560546875, 0.68084716796875, 0.66876220703125, 0.69488525390625, 0.66790771484375, 0.69207763671875, 0.67999267578125, 0.65826416015625, 0.67266845703125, 0.68902587890625, 0.67706298828125, 0.70941162109375, 0.68646240234375, 0.67706298828125, 0.70892333984375, 0.70477294921875, 0.69927978515625, 0.69427490234375, 0.66546630859375, 0.67193603515625, 0.68695068359375, 0.66497802734375, 0.68951416015625, 0.67596435546875, 0.67169189453125, 0.68572998046875, 0.70245361328125, 0.71160888671875, 0.70135498046875, 0.68768310546875, 0.68316650390625, 0.69927978515625, 0.68255615234375, 0.67059326171875, 0.66436767578125, 0.68243408203125, 0.68072509765625, 0.66998291015625, 0.69219970703125, 0.69378662109375, 0.67706298828125, 0.69427490234375, 0.69268798828125, 0.69805908203125, 0.70050048828125, 0.69818115234375, 0.70123291015625, 0.68853759765625, 0.66046142578125, 0.66766357421875, 0.70794677734375, 0.69207763671875, 0.66644287109375, 0.68316650390625, 0.68414306640625, 0.69537353515625, 0.68670654296875, 0.67449951171875, 0.69500732421875, 0.68853759765625, 0.72869873046875, 0.73480224609375, 0.72735595703125, 0.75091552734375, 0.71405029296875, 0.70135498046875, 0.68634033203125, 0.69097900390625, 0.69854736328125, 0.68975830078125, 0.68060302734375, 0.70794677734375, 0.68060302734375, 0.68719482421875, 0.68011474609375, 0.71160888671875, 0.69769287109375, 0.72027587890625, 0.68841552734375, 0.69500732421875, 0.69317626953125, 0.66900634765625, 0.68121337890625, 0.68206787109375, 0.69427490234375, 0.67132568359375, 0.69195556640625, 0.66143798828125, 0.69671630859375, 0.66400146484375, 0.65533447265625, 0.69268798828125, 0.68157958984375, 0.66400146484375, 0.69439697265625, 0.68365478515625, 0.67987060546875, 0.68548583984375, 0.69110107421875, 0.68157958984375, 0.70318603515625, 0.67425537109375, 0.70111083984375, 0.70513916015625, 0.66961669921875, 0.67926025390625, 0.70098876953125, 0.68438720703125, 0.70050048828125, 0.66571044921875, 0.68194580078125, 0.66998291015625, 0.68121337890625, 0.66400146484375, 0.69598388671875, 0.70465087890625, 0.69500732421875, 0.67620849609375, 0.66241455078125, 0.70782470703125, 0.68853759765625, 0.69329833984375, 0.69207763671875, 0.69927978515625, 0.67803955078125, 0.68304443359375, 0.64556884765625, 0.69842529296875, 0.69476318359375, 0.69793701171875, 0.71636962890625, 0.69561767578125, 0.70916748046875, 0.68365478515625, 0.69000244140625, 0.67987060546875, 0.68560791015625, 0.66168212890625, 0.71331787109375, 0.68988037109375, 0.69805908203125, 0.71832275390625, 0.71368408203125, 0.70855712890625, 0.70037841796875, 0.70538330078125, 0.71026611328125, 0.69842529296875, 0.71356201171875, 0.68963623046875, 0.68634033203125, 0.68353271484375, 0.65045166015625, 0.69195556640625, 0.68597412109375, 0.69903564453125, 0.64508056640625, 0.68951416015625, 0.67620849609375, 0.66693115234375, 0.67071533203125, 0.68804931640625, 0.68829345703125, 0.68743896484375, 0.67474365234375, 0.67999267578125, 0.71124267578125, 0.68475341796875, 0.68426513671875, 0.69586181640625, 0.66656494140625, 0.68853759765625, 0.67669677734375, 0.70404052734375, 0.66070556640625, 0.67864990234375, 0.70330810546875, 0.68157958984375, 0.69854736328125, 0.69854736328125, 0.69207763671875, 0.68963623046875, 0.69110107421875, 0.69110107421875, 0.68280029296875, 0.67364501953125, 0.68927001953125, 0.65985107421875, 0.67095947265625, 0.67962646484375, 0.70086669921875, 0.71356201171875, 0.70184326171875, 0.69622802734375, 0.68646240234375, 0.67291259765625, 0.70428466796875, 0.67987060546875, 0.69500732421875, 0.69989013671875, 0.69757080078125, 0.71466064453125, 0.69586181640625, 0.69158935546875, 0.69915771484375, 0.69488525390625, 0.68048095703125, 0.67608642578125, 0.68658447265625, 0.67132568359375, 0.68914794921875, 0.67376708984375, 0.70404052734375, 0.71575927734375, 0.66839599609375, 0.69049072265625, 0.70819091796875, 0.68621826171875, 0.68341064453125, 0.66632080078125, 0.68109130859375, 0.69366455078125, 0.69976806640625, 0.69158935546875, 0.68560791015625, 0.67767333984375, 0.65753173828125, 0.68975830078125, 0.66973876953125, 0.69244384765625, 0.68328857421875, 0.67950439453125, 0.67974853515625, 0.67340087890625, 0.69512939453125, 0.67303466796875, 0.68060302734375, 0.69451904296875, 0.66973876953125, 0.68035888671875, 0.65240478515625, 0.68194580078125, 0.65887451171875, 0.65887451171875, 0.67108154296875, 0.68255615234375, 0.67767333984375, 0.69451904296875, 0.67401123046875, 0.69561767578125, 0.70709228515625, 0.72369384765625, 0.66607666015625, 0.66619873046875, 0.68853759765625, 0.69146728515625, 0.69329833984375, 0.68841552734375, 0.70538330078125, 0.68524169921875, 0.71807861328125, 0.68450927734375, 0.72247314453125, 0.69818115234375, 0.69964599609375, 0.71588134765625, 0.70965576171875, 0.68597412109375, 0.68536376953125, 0.68389892578125, 0.72259521484375, 0.71343994140625, 0.70526123046875, 0.66107177734375, 0.70819091796875, 0.67474365234375, 0.70037841796875, 0.68450927734375, 0.69671630859375, 0.69012451171875, 0.69427490234375, 0.67535400390625, 0.69293212890625, 0.67254638671875, 0.68927001953125, 0.70709228515625, 0.68829345703125, 0.69683837890625, 0.67755126953125, 0.68585205078125, 0.70025634765625, 0.67449951171875, 0.70355224609375, 0.68316650390625, 0.68072509765625, 0.68719482421875, 0.66912841796875, 0.67120361328125, 0.68316650390625, 0.67425537109375, 0.65753173828125, 0.70745849609375, 0.68658447265625, 0.69500732421875, 0.68792724609375, 0.69976806640625, 0.68438720703125, 0.69085693359375, 0.68292236328125, 0.65557861328125, 0.65020751953125, 0.67584228515625, 0.66351318359375, 0.69525146484375, 0.68560791015625, 0.68768310546875, 0.70220947265625, 0.66168212890625, 0.70159912109375, 0.68438720703125, 0.65985107421875, 0.68780517578125, 0.68450927734375, 0.69696044921875, 0.69989013671875, 0.68170166015625, 0.69219970703125, 0.66400146484375, 0.69366455078125, 0.69219970703125, 0.70367431640625, 0.67193603515625, 0.68060302734375, 0.68927001953125, 0.69952392578125, 0.67755126953125, 0.73175048828125, 0.66082763671875, 0.70989990234375, 0.66363525390625, 0.68438720703125, 0.70245361328125, 0.68414306640625, 0.71551513671875, 0.66961669921875, 0.67327880859375, 0.68829345703125, 0.66986083984375, 0.67254638671875, 0.69891357421875, 0.69610595703125, 0.72406005859375, 0.67657470703125, 0.67120361328125, 0.69549560546875, 0.69097900390625, 0.68804931640625, 0.68341064453125, 0.67022705078125, 0.67071533203125, 0.68145751953125, 0.68572998046875, 0.69781494140625, 0.65301513671875, 0.67071533203125, 0.69781494140625, 0.70819091796875, 0.67291259765625, 0.67926025390625, 0.71295166015625, 0.69244384765625, 0.68353271484375, 0.67462158203125, 0.70379638671875, 0.67840576171875, 0.67462158203125, 0.69354248046875, 0.66986083984375, 0.68304443359375, 0.68328857421875, 0.68768310546875, 0.67083740234375, 0.64532470703125, 0.67901611328125, 0.65313720703125, 0.71148681640625, 0.69696044921875, 0.68682861328125, 0.69012451171875, 0.70025634765625, 0.69866943359375, 0.67132568359375, 0.68560791015625, 0.68792724609375, 0.70013427734375, 0.65875244140625, 0.67474365234375, 0.68414306640625, 0.69793701171875, 0.69366455078125, 0.69537353515625, 0.68804931640625, 0.69940185546875, 0.70269775390625, 0.69256591796875, 0.68951416015625, 0.67535400390625, 0.68597412109375, 0.67108154296875, 0.70135498046875, 0.69244384765625, 0.71075439453125, 0.71221923828125, 0.69940185546875, 0.68475341796875, 0.67559814453125, 0.70758056640625, 0.68145751953125, 0.68646240234375, 0.68389892578125, 0.71490478515625, 0.67364501953125, 0.69476318359375, 0.70257568359375, 0.71417236328125, 0.68389892578125, 0.70880126953125, 0.69024658203125, 0.70477294921875, 0.67730712890625, 0.67803955078125, 0.70086669921875, 0.70233154296875, 0.70281982421875, 0.70086669921875, 0.70281982421875, 0.71453857421875, 0.67901611328125, 0.68109130859375, 0.68756103515625, 0.67340087890625, 0.68206787109375, 0.69659423828125, 0.68463134765625, 0.66571044921875, 0.69415283203125, 0.69097900390625, 0.66253662109375, 0.67144775390625, 0.64849853515625, 0.71331787109375, 0.68255615234375, 0.67095947265625, 0.67559814453125, 0.68804931640625, 0.69830322265625, 0.69024658203125, 0.70977783203125, 0.68988037109375, 0.69537353515625, 0.67864990234375, 0.67974853515625, 0.68206787109375, 0.67376708984375, 0.65362548828125, 0.67327880859375, 0.67230224609375, 0.70257568359375, 0.69219970703125, 0.71026611328125, 0.69000244140625, 0.70123291015625, 0.68280029296875, 0.66827392578125, 0.70794677734375, 0.68267822265625, 0.68487548828125, 0.69793701171875, 0.69085693359375, 0.67962646484375, 0.70562744140625, 0.71185302734375, 0.68719482421875, 0.70819091796875, 0.68389892578125, 0.69012451171875, 0.69476318359375, 0.69049072265625, 0.69927978515625, 0.70648193359375, 0.68170166015625, 0.69952392578125, 0.69256591796875, 0.70977783203125, 0.67974853515625, 0.68157958984375, 0.72381591796875, 0.68548583984375, 0.70867919921875, 0.69879150390625, 0.69256591796875, 0.68780517578125, 0.69818115234375, 0.71270751953125, 0.70477294921875, 0.71624755859375, 0.70489501953125, 0.72149658203125, 0.70404052734375, 0.67718505859375, 0.67950439453125, 0.71343994140625, 0.68304443359375, 0.70904541015625, 0.67120361328125, 0.68023681640625, 0.68536376953125, 0.68695068359375, 0.67681884765625, 0.69342041015625, 0.66986083984375, 0.68621826171875, 0.67828369140625, 0.70172119140625, 0.67938232421875, 0.66448974609375, 0.70050048828125, 0.68597412109375, 0.69183349609375, 0.69122314453125, 0.67633056640625, 0.66302490234375, 0.67608642578125, 0.66387939453125, 0.68963623046875, 0.70379638671875, 0.68438720703125, 0.69500732421875, 0.68963623046875, 0.69793701171875, 0.67657470703125, 0.69195556640625, 0.68524169921875, 0.68865966796875, 0.69293212890625, 0.69830322265625, 0.69793701171875, 0.68707275390625, 0.68853759765625, 0.69256591796875, 0.69110107421875, 0.71405029296875, 0.69219970703125, 0.69110107421875, 0.67572021484375, 0.70404052734375, 0.70806884765625, 0.69940185546875, 0.69671630859375, 0.69329833984375, 0.69146728515625, 0.69671630859375, 0.68817138671875, 0.70574951171875, 0.73089599609375, 0.67999267578125, 0.70184326171875, 0.68572998046875, 0.71173095703125, 0.69525146484375, 0.70660400390625, 0.69671630859375, 0.66253662109375, 0.67193603515625, 0.69891357421875, 0.69390869140625, 0.70489501953125, 0.68096923828125, 0.69781494140625, 0.67559814453125, 0.69879150390625, 0.66986083984375, 0.72210693359375, 0.68341064453125, 0.68280029296875, 0.66192626953125, 0.68524169921875, 0.66864013671875, 0.67218017578125, 0.69329833984375, 0.68914794921875, 0.67816162109375, 0.66241455078125, 0.68133544921875, 0.66680908203125, 0.70697021484375, 0.66607666015625, 0.67950439453125, 0.68548583984375, 0.68328857421875, 0.68682861328125, 0.69464111328125, 0.70037841796875, 0.68267822265625, 0.68377685546875, 0.68316650390625, 0.68780517578125, 0.68890380859375, 0.66180419921875, 0.67291259765625, 0.67584228515625, 0.72296142578125, 0.69708251953125, 0.68414306640625, 0.68682861328125, 0.68109130859375, 0.69866943359375, 0.67803955078125, 0.69012451171875, 0.69635009765625, 0.68426513671875, 0.67889404296875, 0.67742919921875, 0.68914794921875, 0.69647216796875, 0.71612548828125, 0.69952392578125, 0.69598388671875, 0.65814208984375, 0.72039794921875, 0.66278076171875, 0.68487548828125, 0.68695068359375, 0.71649169921875, 0.69464111328125, 0.68194580078125, 0.69415283203125, 0.67462158203125, 0.67340087890625, 0.69586181640625, 0.69293212890625, 0.69781494140625, 0.68218994140625, 0.70916748046875, 0.70404052734375, 0.69915771484375, 0.69256591796875, 0.65350341796875, 0.67230224609375, 0.68353271484375, 0.70294189453125, 0.70819091796875, 0.66912841796875, 0.65509033203125, 0.68023681640625, 0.69219970703125, 0.69219970703125, 0.66998291015625, 0.67279052734375, 0.68267822265625, 0.67852783203125, 0.70721435546875, 0.65362548828125, 0.69000244140625, 0.67254638671875, 0.66485595703125, 0.68328857421875, 0.69207763671875, 0.65948486328125, 0.69952392578125, 0.65582275390625, 0.65850830078125, 0.67913818359375, 0.65728759765625, 0.67437744140625, 0.68780517578125, 0.69842529296875, 0.69366455078125, 0.68731689453125, 0.68743896484375, 0.69818115234375, 0.70660400390625, 0.66864013671875, 0.69378662109375, 0.70306396484375, 0.69586181640625, 0.68145751953125, 0.67864990234375, 0.68450927734375, 0.70806884765625, 0.69451904296875, 0.69024658203125, 0.67327880859375, 0.68719482421875, 0.67901611328125, 0.69415283203125, 0.69073486328125, 0.68280029296875, 0.69549560546875, 0.67205810546875, 0.67376708984375, 0.67938232421875, 0.67218017578125, 0.70977783203125, 0.68621826171875, 0.69097900390625, 0.67291259765625, 0.70050048828125, 0.66876220703125, 0.71295166015625, 0.68316650390625, 0.69171142578125, 0.67108154296875, 0.69317626953125, 0.70855712890625, 0.69146728515625, 0.68670654296875, 0.70416259765625, 0.70611572265625, 0.69696044921875, 0.68011474609375, 0.66680908203125, 0.67462158203125, 0.69537353515625, 0.69598388671875, 0.72369384765625, 0.68280029296875, 0.69879150390625, 0.69537353515625, 0.70001220703125, 0.68182373046875, 0.70172119140625, 0.68438720703125, 0.67864990234375, 0.69940185546875, 0.71380615234375, 0.68756103515625, 0.68597412109375, 0.69244384765625, 0.70172119140625, 0.72320556640625, 0.70648193359375, 0.70465087890625, 0.67572021484375, 0.68927001953125, 0.68353271484375, 0.68841552734375, 0.68023681640625, 0.66192626953125, 0.68353271484375, 0.69757080078125, 0.67938232421875, 0.66754150390625, 0.64996337890625, 0.69769287109375, 0.65887451171875, 0.69744873046875, 0.68426513671875, 0.70989990234375, 0.69903564453125, 0.69293212890625, 0.71734619140625, 0.68963623046875, 0.67376708984375, 0.66937255859375, 0.70013427734375, 0.69708251953125, 0.70245361328125, 0.70867919921875, 0.69256591796875, 0.71063232421875, 0.71258544921875, 0.67840576171875, 0.70416259765625, 0.70501708984375, 0.66156005859375, 0.69232177734375, 0.68231201171875, 0.71221923828125, 0.68890380859375, 0.68634033203125, 0.69232177734375, 0.68682861328125, 0.70404052734375, 0.69036865234375, 0.66131591796875, 0.66632080078125, 0.67193603515625, 0.68450927734375, 0.72174072265625, 0.67681884765625, 0.73175048828125, 0.71087646484375, 0.72320556640625, 0.72540283203125, 0.70245361328125, 0.68218994140625, 0.69232177734375, 0.69732666015625, 0.67974853515625, 0.68853759765625, 0.68682861328125, 0.69085693359375, 0.67510986328125, 0.70123291015625, 0.68304443359375, 0.70465087890625, 0.67803955078125, 0.69122314453125, 0.70172119140625, 0.68695068359375, 0.67620849609375, 0.67462158203125, 0.68951416015625, 0.68487548828125, 0.71820068359375, 0.67022705078125, 0.68536376953125, 0.69598388671875, 0.67950439453125, 0.68707275390625, 0.67987060546875, 0.67181396484375, 0.67755126953125, 0.69268798828125, 0.68572998046875, 0.69183349609375, 0.69500732421875, 0.69110107421875, 0.69036865234375, 0.68951416015625, 0.67449951171875, 0.69573974609375, 0.66448974609375, 0.67694091796875, 0.70477294921875, 0.68475341796875, 0.70941162109375, 0.69171142578125, 0.67779541015625, 0.69903564453125, 0.67218017578125, 0.69769287109375, 0.68524169921875, 0.67083740234375, 0.70379638671875, 0.70440673828125, 0.71136474609375, 0.70709228515625, 0.73529052734375, 0.69903564453125, 0.72003173828125, 0.67340087890625, 0.69110107421875, 0.68548583984375, 0.70111083984375, 0.69061279296875, 0.66986083984375, 0.69537353515625, 0.70318603515625, 0.67340087890625, 0.70074462890625, 0.69305419921875, 0.68304443359375, 0.68963623046875, 0.67669677734375, 0.68963623046875, 0.67083740234375, 0.69488525390625, 0.68182373046875, 0.67718505859375, 0.68011474609375, 0.69732666015625, 0.68670654296875, 0.67071533203125, 0.69622802734375, 0.66302490234375, 0.69146728515625, 0.67486572265625, 0.66558837890625, 0.64764404296875, 0.68572998046875, 0.67987060546875, 0.66510009765625, 0.69354248046875, 0.70574951171875, 0.68597412109375, 0.69049072265625, 0.65423583984375, 0.65557861328125, 0.65643310546875, 0.67425537109375, 0.67803955078125, 0.66973876953125, 0.70086669921875, 0.67230224609375, 0.66546630859375, 0.69769287109375, 0.68218994140625, 0.69244384765625, 0.68365478515625, 0.69134521484375, 0.66949462890625, 0.70550537109375, 0.69366455078125, 0.70843505859375, 0.65289306640625, 0.70489501953125, 0.69708251953125, 0.69927978515625, 0.70025634765625, 0.70965576171875, 0.68939208984375, 0.69281005859375, 0.70721435546875, 0.70318603515625, 0.67950439453125, 0.69866943359375, 0.69305419921875, 0.69097900390625, 0.69952392578125, 0.69781494140625, 0.70660400390625, 0.69171142578125, 0.69769287109375, 0.68927001953125, 0.66668701171875, 0.69671630859375, 0.68914794921875, 0.69158935546875, 0.70770263671875, 0.72344970703125, 0.67352294921875, 0.68511962890625, 0.68170166015625, 0.66864013671875, 0.67633056640625, 0.69805908203125, 0.66082763671875, 0.67388916015625, 0.68731689453125, 0.67657470703125, 0.67523193359375, 0.68170166015625, 0.65350341796875, 0.70709228515625, 0.65509033203125, 0.66473388671875, 0.69415283203125, 0.71881103515625, 0.70391845703125, 0.66375732421875, 0.67803955078125, 0.67657470703125, 0.70147705078125, 0.69805908203125, 0.70001220703125, 0.68389892578125, 0.67266845703125, 0.67047119140625, 0.68865966796875, 0.66400146484375, 0.68829345703125, 0.67279052734375, 0.68280029296875, 0.70477294921875, 0.67340087890625, 0.70269775390625, 0.67840576171875, 0.69073486328125, 0.68011474609375, 0.72430419921875, 0.67059326171875, 0.67913818359375, 0.67938232421875, 0.67987060546875, 0.67584228515625, 0.70159912109375, 0.66815185546875, 0.68365478515625, 0.69390869140625, 0.69573974609375, 0.70233154296875, 0.68572998046875, 0.67657470703125, 0.68218994140625, 0.70013427734375, 0.69000244140625, 0.65521240234375, 0.67230224609375, 0.67864990234375, 0.68585205078125, 0.69671630859375, 0.69842529296875, 0.67633056640625, 0.70550537109375, 0.68646240234375, 0.69866943359375, 0.68878173828125, 0.66961669921875, 0.68170166015625, 0.67449951171875, 0.68316650390625, 0.69378662109375, 0.69500732421875, 0.69671630859375, 0.66998291015625, 0.71844482421875, 0.65960693359375, 0.67242431640625, 0.66204833984375, 0.68927001953125, 0.68841552734375, 0.70404052734375, 0.70489501953125, 0.69842529296875, 0.71270751953125, 0.70611572265625, 0.66876220703125, 0.68292236328125, 0.70452880859375, 0.68511962890625, 0.68328857421875, 0.69036865234375, 0.66607666015625, 0.69134521484375, 0.71392822265625, 0.67144775390625, 0.70770263671875, 0.71051025390625, 0.68768310546875, 0.68365478515625, 0.69219970703125, 0.69537353515625, 0.68939208984375, 0.70428466796875, 0.67926025390625, 0.69024658203125, 0.70306396484375, 0.66986083984375, 0.69561767578125, 0.69232177734375, 0.70831298828125, 0.67156982421875, 0.65631103515625, 0.70867919921875, 0.67449951171875, 0.68438720703125, 0.65753173828125, 0.71002197265625, 0.67669677734375, 0.71551513671875, 0.67596435546875, 0.69281005859375, 0.69488525390625, 0.68463134765625, 0.68865966796875, 0.68328857421875, 0.71051025390625, 0.71417236328125, 0.70587158203125, 0.66033935546875, 0.71722412109375, 0.69464111328125, 0.68524169921875, 0.67877197265625, 0.68475341796875, 0.66656494140625, 0.67694091796875, 0.70977783203125, 0.71478271484375, 0.69854736328125, 0.68109130859375, 0.69244384765625, 0.70904541015625, 0.68353271484375, 0.70233154296875, 0.66864013671875, 0.70281982421875, 0.69451904296875, 0.69378662109375, 0.68572998046875, 0.70648193359375, 0.68988037109375, 0.71917724609375, 0.70416259765625, 0.69598388671875, 0.67999267578125, 0.67376708984375, 0.70623779296875, 0.66778564453125, 0.67047119140625, 0.69378662109375, 0.71929931640625, 0.68841552734375, 0.69732666015625, 0.67462158203125, 0.68670654296875, 0.70013427734375, 0.68524169921875, 0.67181396484375, 0.67352294921875, 0.69769287109375, 0.68780517578125, 0.68170166015625, 0.68524169921875, 0.67486572265625, 0.68524169921875, 0.65386962890625, 0.62579345703125, 0.65704345703125, 0.64813232421875, 0.66741943359375, 0.68353271484375, 0.67999267578125, 0.69830322265625, 0.67791748046875, 0.69146728515625, 0.70184326171875, 0.67803955078125, 0.69110107421875, 0.67974853515625, 0.69049072265625, 0.65777587890625, 0.66070556640625, 0.69207763671875, 0.68646240234375, 0.64691162109375, 0.67327880859375, 0.68377685546875, 0.66815185546875, 0.70098876953125, 0.69598388671875, 0.70501708984375, 0.66815185546875, 0.70501708984375, 0.68218994140625, 0.69061279296875, 0.68511962890625, 0.68988037109375, 0.70611572265625, 0.67254638671875, 0.69036865234375, 0.68548583984375, 0.70098876953125, 0.71112060546875, 0.69366455078125, 0.67999267578125, 0.69464111328125, 0.70355224609375, 0.70465087890625, 0.69158935546875, 0.69158935546875, 0.69146728515625, 0.66314697265625, 0.67120361328125, 0.69451904296875, 0.68609619140625, 0.68438720703125, 0.66143798828125, 0.69952392578125, 0.70880126953125, 0.68157958984375, 0.69891357421875, 0.68658447265625, 0.67828369140625, 0.68792724609375, 0.69476318359375, 0.66668701171875, 0.67071533203125, 0.66265869140625, 0.69329833984375, 0.69158935546875, 0.68109130859375, 0.66192626953125, 0.69293212890625, 0.68121337890625, 0.69329833984375, 0.67242431640625, 0.67974853515625, 0.67938232421875, 0.69268798828125, 0.67132568359375, 0.68365478515625, 0.71514892578125, 0.67474365234375, 0.68487548828125, 0.70220947265625, 0.70477294921875, 0.66522216796875, 0.70111083984375, 0.68389892578125, 0.68243408203125, 0.69586181640625, 0.68585205078125, 0.67449951171875, 0.68829345703125, 0.70147705078125, 0.69012451171875, 0.70819091796875, 0.69390869140625, 0.67132568359375, 0.68011474609375, 0.66009521484375, 0.69427490234375, 0.68450927734375, 0.69757080078125, 0.69268798828125, 0.69293212890625, 0.67242431640625, 0.71002197265625, 0.67852783203125, 0.70709228515625, 0.70635986328125, 0.68109130859375, 0.66461181640625, 0.70355224609375, 0.70977783203125, 0.68878173828125, 0.69256591796875, 0.69073486328125, 0.70111083984375, 0.68414306640625, 0.69903564453125, 0.68865966796875, 0.68109130859375, 0.68292236328125, 0.66375732421875, 0.65899658203125, 0.69805908203125, 0.69049072265625, 0.68084716796875, 0.67132568359375, 0.66094970703125, 0.66851806640625, 0.68951416015625, 0.68841552734375, 0.67828369140625, 0.69049072265625, 0.67840576171875, 0.68609619140625, 0.64788818359375, 0.67413330078125, 0.67266845703125, 0.69696044921875, 0.68438720703125, 0.66461181640625, 0.68963623046875, 0.67694091796875, 0.69305419921875, 0.70538330078125, 0.69439697265625, 0.65802001953125, 0.69476318359375, 0.70684814453125, 0.67987060546875, 0.69744873046875, 0.71783447265625, 0.69415283203125, 0.67034912109375, 0.71942138671875, 0.68450927734375, 0.70721435546875, 0.68707275390625, 0.67425537109375, 0.69293212890625, 0.67950439453125, 0.70758056640625, 0.69268798828125, 0.70037841796875, 0.69171142578125, 0.67840576171875, 0.69061279296875, 0.70745849609375, 0.68499755859375, 0.69049072265625, 0.69647216796875, 0.66949462890625, 0.68572998046875, 0.68182373046875, 0.68182373046875, 0.71868896484375, 0.67205810546875, 0.66192626953125, 0.70245361328125, 0.71368408203125, 0.69268798828125, 0.66925048828125, 0.69573974609375, 0.68597412109375, 0.67498779296875, 0.69793701171875, 0.65936279296875, 0.70208740234375, 0.70635986328125, 0.71636962890625, 0.69390869140625, 0.68096923828125, 0.69805908203125, 0.71929931640625, 0.69683837890625, 0.68402099609375, 0.68450927734375, 0.66046142578125, 0.68682861328125, 0.68023681640625, 0.67291259765625, 0.68475341796875, 0.69036865234375, 0.66986083984375, 0.69268798828125, 0.67498779296875, 0.68511962890625, 0.66729736328125]] ("Array"), create if not found? (T)=TRUE) -> (queue out=w20:refnum<queue>, error out=w15:errorcluster)  [unwired: 1 in, 1 out]
  n18 = Obtain Queue(name (unnamed)="GAge Satus", element data type=VIstatus."single acquire" ("VI status")) -> (queue out=w7:refnum<queue>, error out=w25:errorcluster)  [unwired: 3 in, 1 out]
  n19 = Obtain Queue(name (unnamed)="stream queue", element data type=T11 {"Command/Status"="", "Data"=variant, "Session Hash"=0, "Sequence Number"=0} ("NetworkStreamCluster")) -> (queue out=w10:refnum<queue>, error out=w8:errorcluster)  [unwired: 3 in, 1 out]
  n20 = while {
    tunnel: w28 -> [w62]
    tunnel: [w61] -> w27
    tunnel: w7 -> [w67]
    shift-right: [w56] -> _
    shift-left: w22 -> [w60]
    tunnel: w20 -> [w52]
    stop <- w65 stop-if-true
    w54 = VIstatus."stop VI" ("VI status")
    # "Gage status loop"
    n21 = Get Queue Status(queue=w67, return elements? (F)=TRUE) -> (queue out=w63:refnum<queue>, error out=w55:errorcluster, elements=w66:T1[])  [unwired: 1 in, 5 out]
    n22 = Index Array(array=w66, index=0) -> (element=w57:T1)
    n23 = Equal?(x=w57, y=w54) -> (x = y?=w58:bool)
    n24 = Select(t=w54, s=w58, f=w60) -> (s? t:f=w53:T1)
    "loop status" <- w53
    n25 = case shown="\"single acquire\"" w53 {
      tunnel: [FALSE FALSE TRUE FALSE _] -> w65
      tunnel: [w72 w81 w105 w115 _] -> _
      tunnel: w63 -> [w73 w81 w105 w115 _]
      tunnel: w62 -> [w74 w80 w104 w113 w162]
      tunnel: [w74 w77 w104 w108 w159] -> w61
      tunnel: [w71 VIstatus."wait" ("VI status") VIstatus."stop VI" ("VI status") w110 w163] -> w56
      tunnel: w55 -> [w70 w79 w103 w114 _]
      tunnel: [w69 w79 w103 w114 _] -> _
      tunnel: w52 -> [_ _ _ _ w157]
      frame "busy", Default {
        n26 = Dequeue Element(queue=w73, error in (no error)=w70) -> (queue out=w72:refnum<queue>, element=w71:T1, error out=w69:errorcluster)  [unwired: 1 in, 1 out]
      }
      frame "update config" {
        n27 = flat-sequence {
          tunnel: w80 -> [w90]
          tunnel: [w83] -> w78
          tunnel: ["Acquisition"] -> w76
          tunnel: [w101] -> w77
          tunnel: w78 -> [w101]
          tunnel: w76 -> [w100]
          frame #0 {
            n28 = call "ConfigureAquisition.vi"("Acquisition"="Acquisition", "Trigger"="Trigger", "channels configuration"="channels \nconfiguration", "Handle Cluster"=w90) -> ("Handle Cluster 2"=w83:T4)  [unwired: 6 in, 1 out]
            n29 = call <userlib>:"CsTool-Commit.vi"("Coerce Flag (f)"=TRUE, "Handle Cluster"=w83) -> ("Error Code"=w86:i32)  [unwired: 1 in, 1 out]
            n30 = call <userlib>:"CsTool-ErrorHandler.vi"("StopOnError (true)"=TRUE, "Error Code"=w86, "Handle Cluster"=w83) -> ()  [unwired: 1 out]
          }
          frame #1 {
            n31 = call <userlib>:"CsTool-QueryAcquisitionParameters.vi"("Handle Cluster"=w101) -> ("Trigger Delay"=w96:dbl, "Trigger Holdoff"=w95:dbl, "Trigger Timeout"=w94:dbl, "Depth"=w97:dbl, "Segment Count"=w91:u32, "Segment Size"=w93:dbl, "Clock Mode"=w98:enum16{"Internal", "External", "Reference"}, "Sample Rate"=w99:dbl)  [unwired: 3 out]
            n32 = Bundle By Name(cluster=w100, "averaging"=w91, "Segment Size"=w93, "Trigger Timeout"=w94, "Trigger Holdoff"=w95, "Trigger Delay"=w96, "post trigger"=w97, "Clock mode"=w98, "Sample Rate"=w99) -> (w92:T8)
            "current aquisition" <- w92
            n33 = property on="Acquisition" class="Clust (strict)"("Value"=w92) -> ()  [unwired: 2 in, 2 out]
          }
        }
      }
      frame "stop VI" {
      }
      frame "single acquire" {
        n34 = flat-sequence {
          tunnel: w113 -> [w121]
          tunnel: [w121] -> w112
          tunnel: w112 -> [w123]
          tunnel: [w123] -> w111
          tunnel: w111 -> [w150]
          tunnel: [w150] -> w109
          frame #0 {
            # "start aquisition"
            n35 = call <userlib>:"CsTool-Capture.vi"("Handle Cluster"=w121) -> ("Error Code"=w122:i32)
            n36 = call <userlib>:"CsTool-ErrorHandler.vi"("Error Code"=w122, "Handle Cluster"=w121) -> ()  [unwired: 1 in, 1 out]
          }
          frame #1 {
            # "wait for aquisition to finish"
            n37 = while {
              tunnel: w123 -> [w128]
              shift-right: [w126] -> _
              shift-left: _ -> [w125]
              stop <- w127 stop-if-true
              n38 = flat-sequence {
                tunnel: [w134] -> w130
                tunnel: w128 -> [w133]
                tunnel: w125 -> [w131]
                tunnel: [w131] -> w124
                tunnel: [w142] -> w126
                tunnel: w124 -> [w143]
                frame #0 {
                  n39 = call <userlib>:"CsTool-QueryStatus.vi"("Handle Cluster"=w133) -> ("Status"=w134:i32)
                  n40 = case shown="0" w134 {
                    tunnel: ["Ready" "Waiting" "Triggered" "Transferring" "Calibrating" " "] -> w132
                    frame 0 {
                    }
                    frame 1 {
                    }
                    frame 2 {
                    }
                    frame 3 {
                    }
                    frame 4 {
                    }
                    frame 5, Default {
                    }
                  }
                  n41 = property on="Gage progess" class="Str"("Value"=w132) -> ()  [unwired: 2 in, 2 out]
                }
                frame #1 {
                  n42 = Tick Count (ms)() -> (millisecond timer value=w142:u32)
                  n43 = Subtract(x=w142, y=w143) -> (x-y=→"aquire time (ms)":u32)
                }
              }
              n44 = Equal?(x=w130, y=0) -> (x = y?=w127:bool)
            }
            "Handle Cluster" <- w123
          }
          frame #2 {
            # "channel 1 : \"0\""
            # "transfers data to labview"
            n45 = property on="current aquisition" class="Clust (strict)"() -> ("Value"=w147:T3)  [unwired: 2 in, 2 out]
            n46 = Unbundle By Name(w147) -> ("number of records"=w148:u32, "Mode"=w146:u16)  [unwired: 1 out]
            n47 = case shown="1, Default" w146 {
              tunnel: [1 4] -> w149
              frame 1, Default {
              }
              frame 2 {
              }
            }
            n48 = for {
              N: w149 -> [_]
              tunnel: w150 -> [w156]
              tunnel: w148 -> [w154]
              tunnel: [w153] -> w145 mode=indexing
              i -> [w155]
              # "loop on channels\n(usually only 1)"
              n49 = call "TransferSegments.vi"("segment number"=w154, "Channel (0)"=w155, "Handle Cluster"=w156) -> ("Data in Volts"=w153:dbl[][])  [unwired: 7 in, 1 out]
            }
            n50 = call "AverageSignal.vi"("Data in Volts"=w145) -> ("Array"=→"Waveform Graph":dbl[][])  [unwired: 10 in]
          }
        }
        n51 = case shown="False" "Continuous" {
          tunnel: [VIstatus."wait" ("VI status") VIstatus."single acquire" ("VI status")] -> w110
          tunnel: w109 -> [w118 w120]
          tunnel: [w118 w120] -> w108
          frame False {
          }
          frame True {
          }
        }
      }
      frame "loop acquire" {
        n52 = flat-sequence {
          tunnel: w162 -> [w164]
          tunnel: [w164] -> w161
          tunnel: w161 -> [w166]
          tunnel: [w166] -> w160
          tunnel: [w184] -> w159
          tunnel: w160 -> [w184]
          tunnel: w157 -> [w178]
          frame #0 {
            # "intit acquire"
            n53 = call <userlib>:"CsTool-Capture.vi"("Handle Cluster"=w164) -> ("Error Code"=w165:i32)
            n54 = call <userlib>:"CsTool-ErrorHandler.vi"("Error Code"=w165, "Handle Cluster"=w164) -> ()  [unwired: 1 in, 1 out]
          }
          frame #1 {
            # "acquire on averaging number"
            n55 = while {
              tunnel: w166 -> [w171]
              stop <- w167 stop-if-true
              n56 = call <userlib>:"CsTool-QueryStatus.vi"("Handle Cluster"=w171) -> ("Status"=w169:i32)
              n57 = case shown="0" w169 {
                tunnel: ["Ready" "Waiting" "Triggered" "Transferring" "Calibrating" " "] -> w170
                frame 0 {
                }
                frame 1 {
                }
                frame 2 {
                }
                frame 3 {
                }
                frame 4 {
                }
                frame 5, Default {
                }
              }
              n58 = Equal?(x=w169, y=0) -> (x = y?=w167:bool)
              n59 = property on="Gage progess" class="Str"("Value"=w170) -> ()  [unwired: 2 in, 2 out]
            }
          }
          frame #2 {
            # "store data to current data queue"
            n60 = property on="Acquisition" class="Clust (strict)"() -> ("Value"=w183:T8)  [unwired: 2 in, 2 out]
            n61 = Unbundle By Name(w183) -> ("averaging"=w182:u32)
            n62 = for {
              N: 1 -> [_]
              tunnel: w184 -> [w188]
              tunnel: w182 -> [w186]
              tunnel: [w185] -> w181 mode=indexing
              n63 = call "TransferSegments.vi"("segment number"=w186, "Channel (0)"=u16 0, "Handle Cluster"=w188) -> ("Data in Volts"=w185:dbl[][])  [unwired: 7 in, 1 out]
            }
            n64 = call "AverageSignal.vi"("Data in Volts"=w181) -> ("Array"=w179:dbl[][])  [unwired: 10 in]
            n65 = Enqueue Element(queue=w178, element=w179) -> ()  [unwired: 2 in, 3 out]
          }
        }
        n66 = case shown="True" TRUE {
          tunnel: [VIstatus."loop acquire" ("VI status") VIstatus."wait" ("VI status")] -> w163
          frame False {
          }
          frame True {
          }
        }
      }
    }
  }
  n67 = while {
    tunnel: w20 -> [w198]
    tunnel: w15 -> [w197]
    tunnel: [w195] -> w14
    shift-right: [w194] -> _
    shift-left: dbl[][] [] ("Array") -> [w192]
    tunnel: w5 -> [w193]
    stop <- w196 stop-if-true
    # "loop acquire slave"
    n68 = Array Size(array=w192) -> (size(s)=→"size(s)":i32[])
    n69 = event shown="[0] Timeout" {
      selector: _ -> [_ _ _]
      dyn-events: _ -> [_ _ _]
      timeout: 0 -> [_ _ _]
      tunnel: w198 -> [w204 _ w224]
      tunnel: w197 -> [w207 _ _]
      tunnel: [_ _ TRUE] -> w196
      tunnel: [w204 _ w224] -> w195
      tunnel: [w203 dbl[][] [] ("Array") w222] -> w194
      tunnel: w192 -> [w202 w218 w222]
      tunnel: w193 -> [w201 _ w223]
      event Timeout {
        n70 = event-data() -> ()  [unwired: 1 in, 3 out]
        n71 = Dequeue Element(queue=w204, timeout in ms (-1)=100, error in (no error)=w207) -> (element=w205:dbl[][], timed out?=w200:bool)  [unwired: 2 out]
        n72 = case shown="False" w200 {
          tunnel: w205 -> [w209 _]
          tunnel: [w208 w216] -> w203
          tunnel: w202 -> [w210 w216]
          tunnel: w201 -> [w211 _]
          frame False {
            n73 = local read "Network Stream State Indicator"() -> (w212:T2)
            n74 = Insert Into Array(array=w210, new element=w209) -> (w208:dbl[][])  [unwired: 2 in]
            n75 = case shown="\"Connected\"" w212 {
              tunnel: w211 -> [_ w214]
              frame "Waiting for connection", Default {
              }
              frame "Connected" {
                n76 = shared-variable-read(w214) -> (w213:refnum<k21>)  [unwired: 1 in, 3 out]
                n77 = local read "Sequence Number"() -> (w215:i64)
                n78 = call "slavedone.vi"("index"=w215, "shared variable refnum out"=w213) -> ()  [unwired: 9 in, 1 out]
              }
            }
            "Intensity Chart" <- w209
          }
          frame True {
          }
        }
      }
      event "Save Loop acquire": Value Change {
        n79 = event-data() -> ()  [unwired: 1 in, 5 out]
        n80 = property on="Acquisition" class="Clust (strict)"() -> ("Controls[]"=w219:refnum<vi>[])  [unwired: 2 in, 2 out]
        n81 = call "SaveArray.vi"("name or relative path"="file name", "saving folder"="saving folder", "parameters cluster"=w219, "array"=w218) -> ()  [unwired: 7 in, 1 out]
      }
      event "Stop Button": Value Change {
        n82 = event-data() -> ()  [unwired: 1 in, 5 out]
        n83 = Close Variable Connection(11:w223) -> ()  [unwired: 1 in, 1 out]
      }
    }
  }
  n84 = while {
    shift-right: [w233] -> _
    shift-left: T12 {"Network Stream Reader Endpoint"="", "Last Received Sequence Number"=0} ("StateMachineVariable") -> [w235]
    shift-right: [w228] -> _
    shift-left: NetworkStreamReceiverState."Program Start" -> [w234]
    shift-right: [w232] -> _
    shift-left: errorcluster {"status"=FALSE, "code"=0, "source"=""} ("error in (no error)") -> [w230]
    tunnel: w10 -> [w226]
    stop <- w231 stop-if-true
    # "Network Stream Reader loop"
    n85 = case shown="\"Waiting for connection\"" w234 {
      tunnel: [NetworkStreamReceiverState."Waiting for connection" w249 w271 NetworkStreamReceiverState."Waiting for connection" NetworkStreamReceiverState."Exit" NetworkStreamReceiverState."Exit"] -> w229
      tunnel: [w239 w248 w272 w308 w321 w329] -> w232
      tunnel: [w238 w247 w269 w304 w314 w326] -> w233
      tunnel: [_ _ _ _ TRUE _] -> w231
      tunnel: w235 -> [w238 w245 w268 w305 w315 w326]
      tunnel: w230 -> [w239 w244 w267 w307 w316 w327]
      tunnel: w226 -> [_ _ w266 _ _ _]
      frame "Program Start", Default {
      }
      frame "Waiting for connection" {
        w246 = T14 1 items=["allocate as needed", "pre-allocate"] ("element allocation mode")
        w253 = 100  # timeout
        n86 = Create Network Stream Reader Endpoint(5:w253, 6:w246, 7:100 ("reader buffer size"), 8:w244, 9:T11 {"Command/Status"="", "Data"=variant, "Session Hash"=0, "Sequence Number"=0} ("NetworkStreamCluster"), 10:"//localhost:ContinuousScanMain/writer3" ("writer url"), 11:"//localhost:Oscilloscope/reader" ("reader name")) -> (0:w250:errorcluster, 3:w242:refnum<k21>)
        n87 = case shown="Error" w250 {
          selector: w250 -> [w254 w257]
          tunnel: [NetworkStreamReceiverState."Connected" w259] -> w249
          tunnel: [w254 w256] -> w248
          frame No Error {
          }
          frame Error {
            n88 = Unbundle By Name(w257) -> ("code"=w258:i32)
            n89 = case shown="-314004" w258 {
              tunnel: [NetworkStreamReceiverState."Unhandled Exception" NetworkStreamReceiverState."Waiting for connection"] -> w259
              tunnel: w257 -> [w260 w263]
              tunnel: [w260 w262] -> w256
              frame 0, Default {
              }
              frame -314004 {
                # "Timed out, try again..."
                n90 = call <vilib>:"Clear Errors.vi"("error in (no error)"=w263, "specific error code to clear (0: all)"=-314004) -> ("error out"=w262:errorcluster)  [unwired: 4 in, 1 out]
              }
            }
          }
        }
        n91 = Bundle By Name(cluster=w245, "Network Stream Reader Endpoint"=w242) -> (w247:T12)
      }
      frame "Connected" {
        n92 = Unbundle By Name(w268) -> ("Network Stream Reader Endpoint"=w270:refnum<k21>)
        n93 = shared-variable-read(w270, w267, 100 ("timeout ms (-1)")) -> (w273:errorcluster, w275:bool, w274:T11)  [unwired: 1 out]
        n94 = case shown="No Error" w273 {
          selector: w273 -> [w282 w301]
          tunnel: w275 -> [w284 _]
          tunnel: w274 -> [w283 _]
          tunnel: [w281 w301] -> w272
          tunnel: [NetworkStreamReceiverState."Connected" w299] -> w271
          tunnel: [w279 w298] -> w269
          tunnel: w268 -> [w278 w298]
          tunnel: w266 -> [w277 _]
          frame No Error {
            n95 = case shown="False" w284 {
              tunnel: [w291 w297] -> w281
              tunnel: w282 -> [w291 w297]
              tunnel: w283 -> [w295 _]
              tunnel: [w292 w296] -> w279
              tunnel: w278 -> [w292 w296]
              tunnel: w277 -> [w290 _]
              frame False {
                n96 = Unbundle By Name(w295) -> ("Session Hash"=w287:u64, "Sequence Number"=w286:u64, "Command/Status"=w294:string, "Data"=w293:variant)
                "Session Hash" <- w287
                n97 = Bundle(cluster=T11 {"Command/Status"="", "Data"=variant, "Session Hash"=0, "Sequence Number"=0} ("NetworkStreamCluster"), "Command/Status"=w294, "Data"=w293, "Session Hash"=w287, "Sequence Number"=w286) -> (w289:T11)
                n98 = Enqueue Element(queue=w290, element=w289, timeout in ms (-1)=100) -> ()  [unwired: 1 in, 3 out]
              }
              frame True {
              }
            }
          }
          frame Error {
            n99 = Unbundle By Name(w301) -> ("code"=w300:i32)
            n100 = case shown="0, Default" w300 {
              tunnel: [NetworkStreamReceiverState."Unhandled Exception" NetworkStreamReceiverState."Connection lost"] -> w299
              frame 0, Default {
              }
              frame -314310, -314220 {
                # "The remote endpoint has been destroyed."
              }
            }
          }
        }
      }
      frame "Connection lost" {
        w311 = refnum<k21> refnum  # reader endpoint
        n101 = Unbundle By Name(w305) -> ("Network Stream Reader Endpoint"=w306:refnum<k21>)
        n102 = Destroy Stream Endpoint(8:w307, 11:w306) -> (0:w310:errorcluster)
        n103 = Bundle By Name(cluster=w305, "Network Stream Reader Endpoint"=w311) -> (w304:T12)
        n104 = call <vilib>:"Clear Errors.vi"("error in (no error)"=w310, "specific error code to clear (0: all)"=0) -> ("error out"=w308:errorcluster)  [unwired: 4 in, 1 out]
      }
      frame "Exit" {
        w317 = refnum<k21> refnum  # reader endpoint
        n105 = Unbundle By Name(w315) -> ("Network Stream Reader Endpoint"=w313:refnum<k21>)
        n106 = Not Equal?(x=w317, y=w313) -> (x != y?=w319:bool)
        n107 = case shown="True" w319 {
          tunnel: [w322 w325] -> w321
          tunnel: w316 -> [w322 w324]
          tunnel: w313 -> [_ w323]
          frame False {
          }
          frame True {
            n108 = Destroy Stream Endpoint(8:w324, 11:w323) -> (0:w325:errorcluster)
          }
        }
        n109 = Bundle By Name(cluster=w315, "Network Stream Reader Endpoint"=w317) -> (w314:T12)
      }
      frame "Unhandled Exception" {
        n110 = call <vilib>:"General Error Handler.vi"("error in (no error)"=w327) -> ("error out"=w329:errorcluster)  [unwired: 10 in, 4 out]
      }
    }
    n111 = Get Queue Status(queue=w226) -> (error out=w227:errorcluster)  [unwired: 2 in, 7 out]
    n112 = case shown="No Error" w227 {
      tunnel: w229 -> [w236 _]
      tunnel: [w236 NetworkStreamReceiverState."Exit"] -> w228
      frame No Error {
      }
      frame Error {
      }
    }
    "Network Stream State Indicator" <- w234
  }
  n113 = while {
    tunnel: w25 -> [w333]
    tunnel: w7 -> [w334]
    tunnel: [w332] -> w24
    tunnel: [w331] -> w23
    stop <- w330 stop-if-true
    # "Command loop for VI"
    n114 = event shown="[4] \"loop acquire\": Value Change" {
      selector: _ -> [_ _ _ _ _]
      dyn-events: _ -> [_ _ _ _ _]
      timeout: _ -> [_ _ _ _ _]
      tunnel: w334 -> [w340 w345 w350 w354 w360]
      tunnel: w333 -> [w339 w342 w348 w355 w357]
      tunnel: [w338 w344 w349 w354 w359] -> w332
      tunnel: [w337 w343 w347 w355 w358] -> w331
      tunnel: [TRUE _ _ _ _] -> w330
      event "Stop Button": Value Change {
        n115 = event-data() -> ()  [unwired: 1 in, 3 out]
        n116 = Enqueue Element(queue=w340, element=VIstatus."stop VI" ("VI status"), error in (no error)=w339) -> (queue out=w338:refnum<queue>, error out=w337:errorcluster)  [unwired: 1 in, 1 out]
      }
      event "configure": Value Change {
        n117 = event-data() -> ()  [unwired: 1 in, 3 out]
        n118 = Enqueue Element(queue=w345, element=VIstatus."update config" ("VI status"), error in (no error)=w342) -> (queue out=w344:refnum<queue>, error out=w343:errorcluster)  [unwired: 1 in, 1 out]
      }
      event "aquire": Value Change {
        n119 = event-data() -> ()  [unwired: 1 in, 3 out]
        n120 = Enqueue Element(queue=w350, element=VIstatus."single acquire" ("VI status"), error in (no error)=w348) -> (queue out=w349:refnum<queue>, error out=w347:errorcluster)  [unwired: 1 in, 1 out]
      }
      event "abort aquisition": Value Change {
        n121 = event-data() -> ()  [unwired: 1 in, 3 out]
        n122 = property on="Handle Cluster" class="Clust (strict)"() -> ("Value"=w352:T4)  [unwired: 2 in, 2 out]
        n123 = call <userlib>:"CsTool-AbortCapture.vi"("Handle Cluster"=w352) -> ("Error Code"=w353:i32)
        n124 = call <userlib>:"CsTool-ErrorHandler.vi"("StopOnError (true)"=TRUE, "Error Code"=w353, "Handle Cluster"=w352) -> ()  [unwired: 1 out]
      }
      event "loop acquire": Value Change {
        n125 = event-data() -> ()  [unwired: 1 in, 3 out]
        n126 = Enqueue Element(queue=w360, element=VIstatus."loop acquire", error in (no error)=w357) -> (queue out=w359:refnum<queue>, error out=w358:errorcluster)  [unwired: 1 in, 1 out]
      }
    }
  }
  n127 = while {
    tunnel: w8 -> [w363]
    tunnel: w10 -> [w364]
    tunnel: w7 -> [w361]
    stop <- w362 stop-if-true
    (unwired) 100 ("timeout in ms (-1)")
    # "Network Stream consumer loop"
    n128 = event shown="[0] Timeout" {
      selector: _ -> [_ _]
      dyn-events: _ -> [_ _]
      timeout: 0 -> [_ _]
      tunnel: w364 -> [w371 w376]
      tunnel: w363 -> [w370 _]
      tunnel: [_ TRUE] -> w362
      tunnel: w361 -> [w366 _]
      event Timeout {
        n129 = event-data() -> ()  [unwired: 1 in, 3 out]
        n130 = Dequeue Element(queue=w371, timeout in ms (-1)=100, error in (no error)=w370) -> (element=w367:T11, timed out?=w368:bool)  [unwired: 2 out]
        n131 = case shown="True" w368 {
          tunnel: w367 -> [w375 _]
          tunnel: w366 -> [w374 _]
          frame False {
            n132 = Unbundle By Name(w375) -> ("Sequence Number"=→"Sequence Number":u64)
            n133 = Enqueue Element(queue=w374, element=VIstatus."loop acquire") -> ()  [unwired: 2 in, 3 out]
          }
          frame True {
          }
        }
      }
      event "Stop Button": Value Change {
        n134 = event-data() -> ()  [unwired: 1 in, 4 out]
        n135 = Release Queue(queue=w376) -> ()  [unwired: 2 in, 3 out]
      }
    }
  }
  n136 = Release Queue(queue=w14) -> (error out=→"error out 2":errorcluster)  [unwired: 2 in, 2 out]
  n137 = flat-sequence {
    tunnel: w27 -> [w381]
    tunnel: w24 -> [w380]
    tunnel: w23 -> [w379]
    frame #0 {
      # "exit and free memory"
      n138 = Release Queue(queue=w380, error in (no error)=w379) -> (error out=→"error out":errorcluster)  [unwired: 1 in, 2 out]
      n139 = call <userlib>:"CsTool-FreeSystem.vi"("Handle Cluster"=w381) -> ()  [unwired: 1 out]
    }
  }
